vi "Main.vi"() -> ()   [LabVIEW 2020]
uses:
  <vilib>/Utility/miscctls.llb/LVBoundsTypeDef.ctl
  <vilib>/Utility/miscctls.llb/LVPointTypeDef.ctl
  <vilib>/Utility/miscctls.llb/LVRangeTypeDef.ctl
  <vilib>/DAQmx/read.llb/DAQmx Read (Analog 1D Wfm NChan NSamp).vi
  <vilib>/Waveform/WDTOps.llb/WDT Append Waveforms DBL.vi
  <vilib>/DAQmx/create/channels.llb/DAQmx Create Channel (AI-Voltage-Basic).vi
  <vilib>/DAQmx/configure/timing.llb/DAQmx Timing (Sample Clock).vi
  <vilib>/DAQmx/miscellaneous.llb/DAQmx Fill In Error Info.vi
  <vilib>/regexp/Match Regular Expression.xnode
  <resource>/objmgr/daqmx.rc
panel:
  out "Counter":dbl
  out "Continious Log Flag":bool
  in  "Continious Log":bool
  in  "Current Amplitude Range":dbl min=1.0 max=200.0 step=1.0
  in  "Voltage Amplitude Range":dbl min=1.0 max=1000.0 step=1.0
  in  "Experiment Name":string
  in  "Level Lower Limit, dB":dbl min=-200.0 max=-10.0 step=10.0
  in  "Freq Upper Limit, Hz":dbl min=0.0 step=1.0
  in  "Freq Lower Limit, Hz":dbl min=0.0 step=1.0
  out "Log flag":bool
  in  "Start Log":bool
  in  "Log length, sec":sgl min=0.2 max=600 step=0.1 format="%.1f"
  out "Current Spectrum":waveform(dbl)[](graph)
  out "Park Spectrum":waveform(dbl)[](graph)
  in  "Park Spectrum Button":bool
  in  "Current Spectrum Button":bool
  in  "Godograph Button":bool
  in  "Voltage Spectrum Button":bool
  in  "Current Button":bool
  in  "Voltage Button":bool
  in  "Plot length , sec":sgl min=0.2 max=60 step=0.1 format="%.1f"
  out "Voltage":waveform(dbl)[](graph)=[{"t0"=timestamp(3706707710.400176 s since 1904-01-01), "dt"=2.4999999999999957e-05, "Y"=array[8000 elements], "attributes"=variant("NI_ChannelName"=variant(string "Voltage A"), "NI_UnitDescription"=variant(string "Volts"))}, {"t0"=timestamp(3706707710.4001803 s since 1904-01-01), "dt"=2.4999999999999957e-05, "Y"=array[8000 elements], "attributes"=variant("NI_ChannelName"=variant(string "Voltage B"), "NI_UnitDescription"=variant(string "Volts"))}, {"t0"=timestamp(3706707710.4001846 s since 1904-01-01), "dt"=2.4999999999999957e-05, "Y"=array[8000 elements], "attributes"=variant("NI_ChannelName"=variant(string "Voltage C"), "NI_UnitDescription"=variant(string "Volts"))}]
  out "Current":waveform(dbl)[](graph)=[{"t0"=timestamp(3706707710.4001637 s since 1904-01-01), "dt"=2.4999999999999957e-05, "Y"=array[8000 elements], "attributes"=variant("NI_ChannelName"=variant(string "Current A"), "NI_UnitDescription"=variant(string "Volts"))}, {"t0"=timestamp(3706707710.400168 s since 1904-01-01), "dt"=2.4999999999999957e-05, "Y"=array[8000 elements], "attributes"=variant("NI_ChannelName"=variant(string "Current B"), "NI_UnitDescription"=variant(string "Volts"))}, {"t0"=timestamp(3706707710.4001718 s since 1904-01-01), "dt"=2.4999999999999957e-05, "Y"=array[8000 elements], "attributes"=variant("NI_ChannelName"=variant(string "Current C"), "NI_UnitDescription"=variant(string "Volts"))}]
  out "Voltage Spectrum":waveform(dbl)[](graph)
  out "Godograph":cluster{"Y":dbl[], "Y":dbl[]}[](graph)
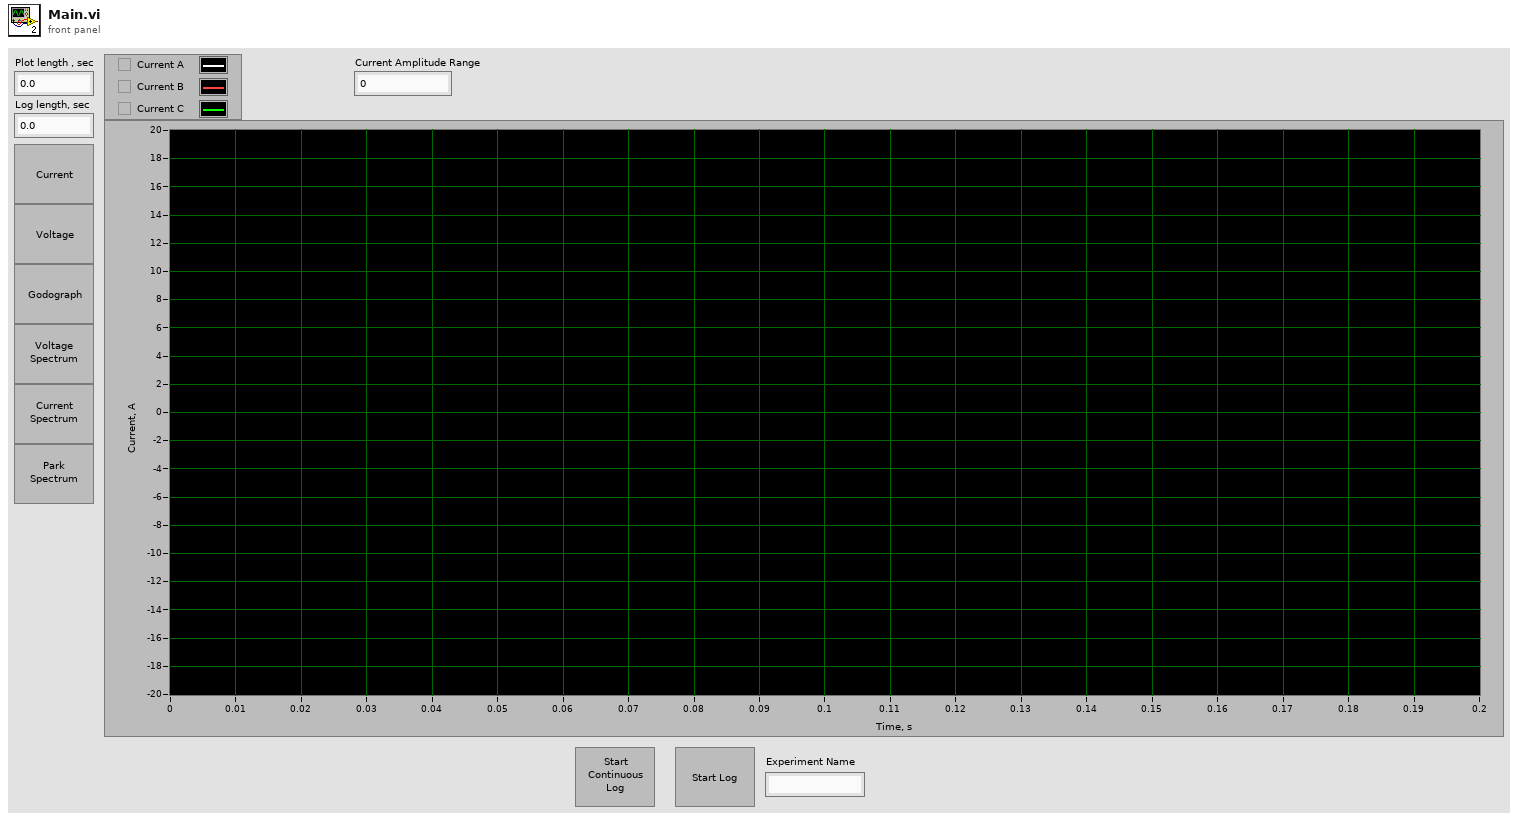
[diagram p1: front panel]
types:
  T1 = typedef "LVBoundsTypeDef.ctl" = cluster{"Width":u32, "Height":u32}
  T2 = typedef "LVPointTypeDef.ctl" = cluster{"Horizontal":i16, "Vertical":i16}
  T3 = enum16{"Always On", "Always Off", "Off While Running"}
  T4 = typedef "LVRangeTypeDef.ctl" = cluster{"Minimum":dbl, "Maximum":dbl, "Increment":dbl, "Minor Increment":dbl, "Start":dbl}
  T5 = enum8{"Enabled", "Disabled", "Disabled and Grayed Out"}
  T6 = enum16{"open", "open or create", "create or replace", "create", "open (read-only)"}
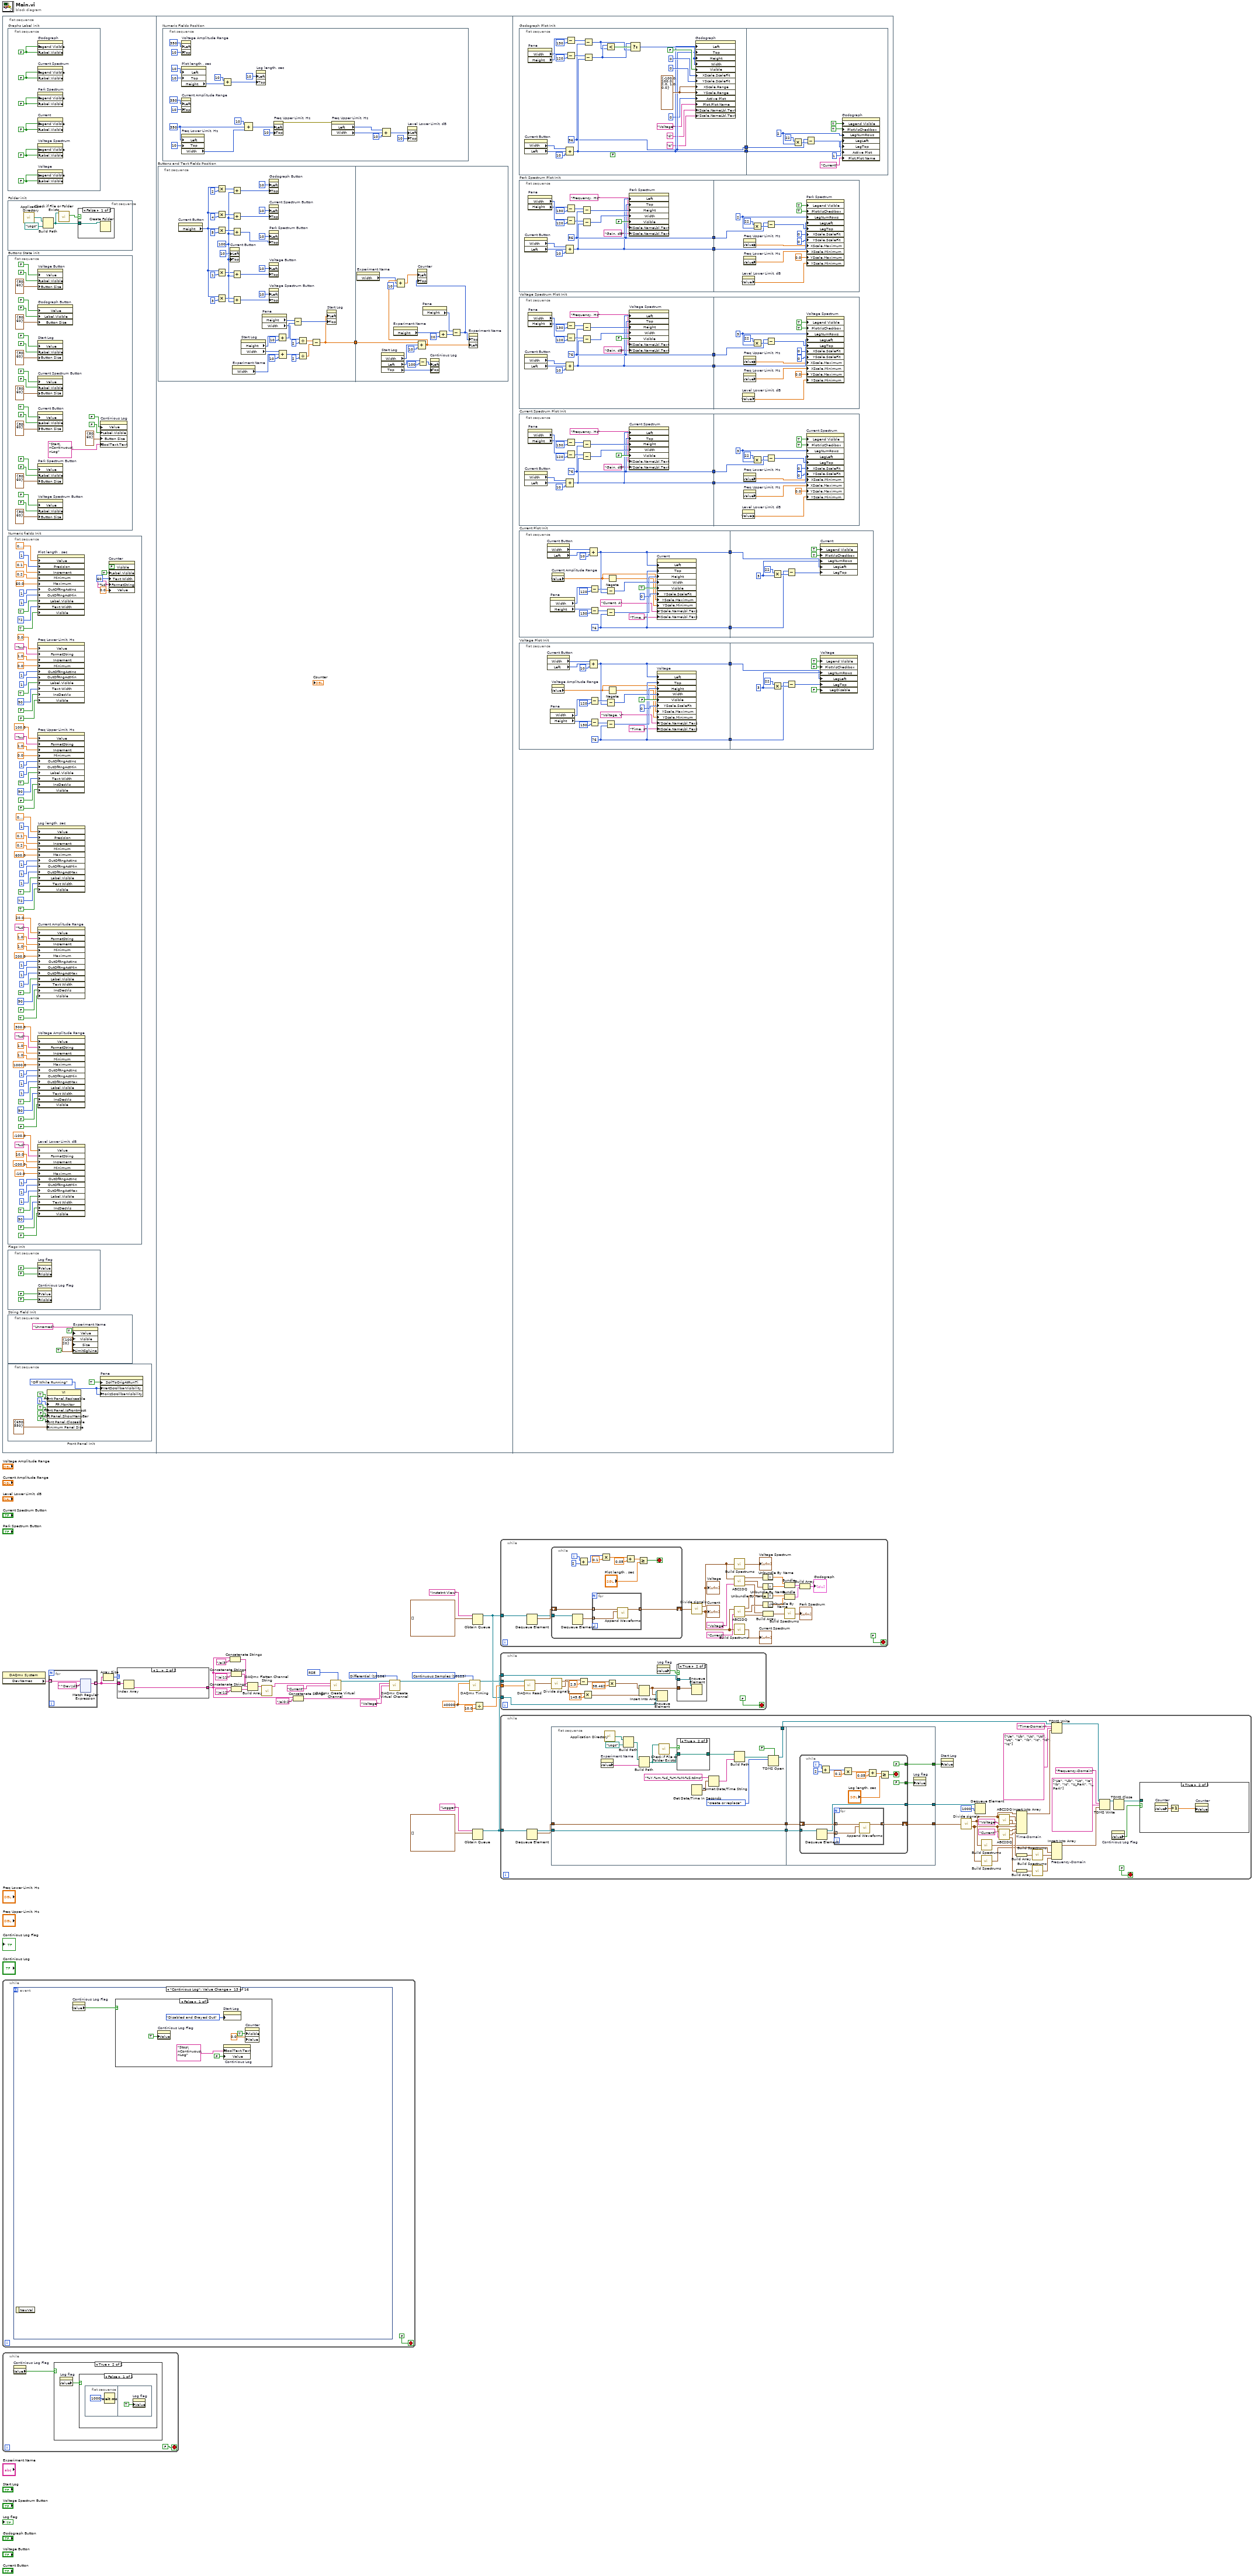
[diagram p0: block diagram]
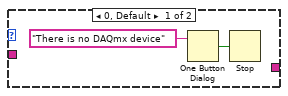
[diagram p2: hidden frame]
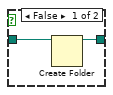
[diagram p6: hidden frame]
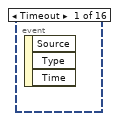
[diagram p8: hidden frame]
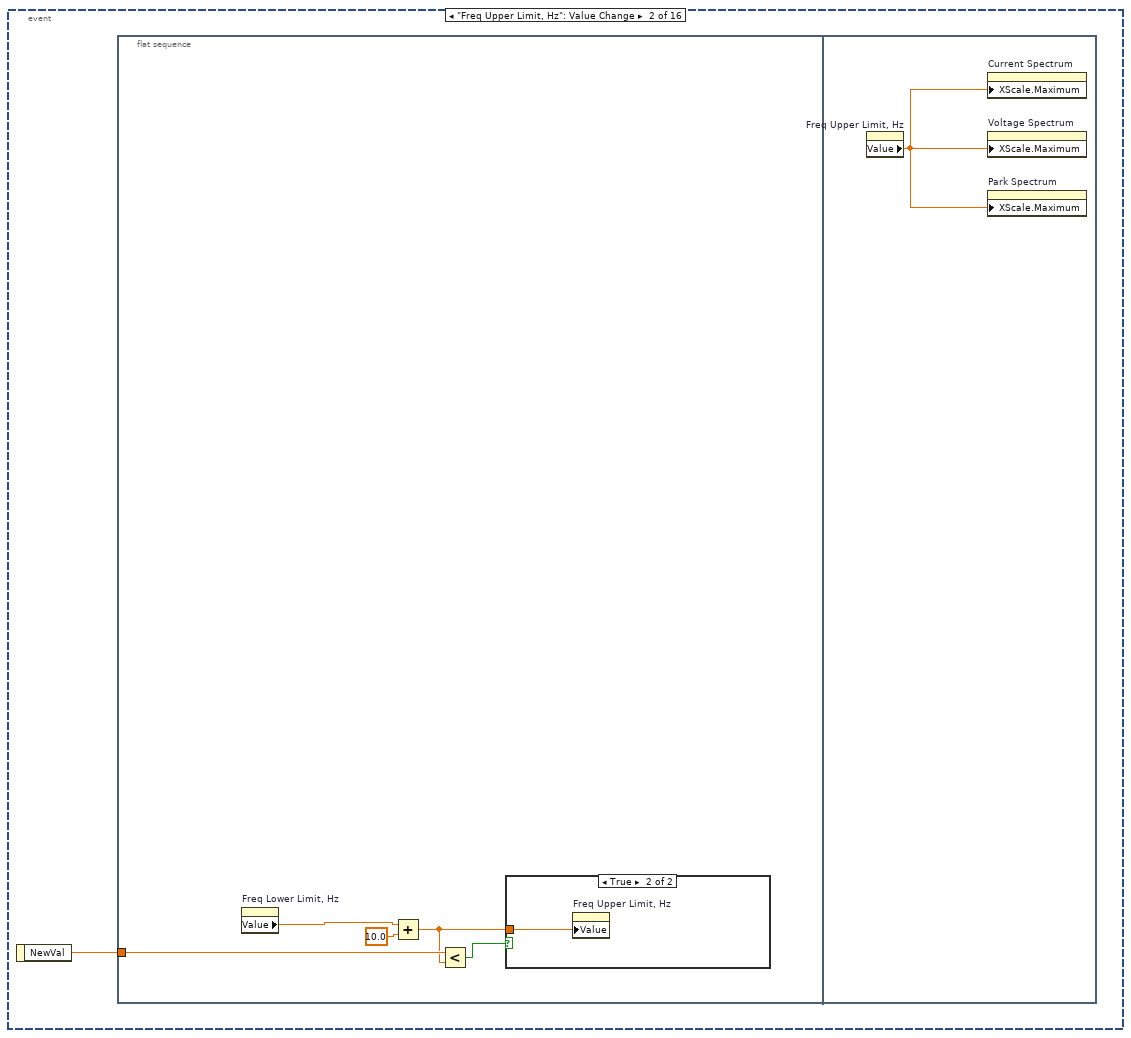
[diagram p9: hidden frame]
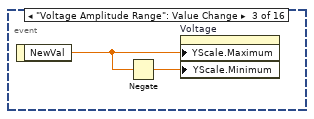
[diagram p11: hidden frame]
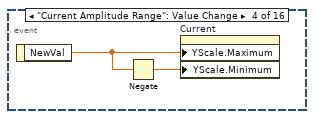
[diagram p12: hidden frame]
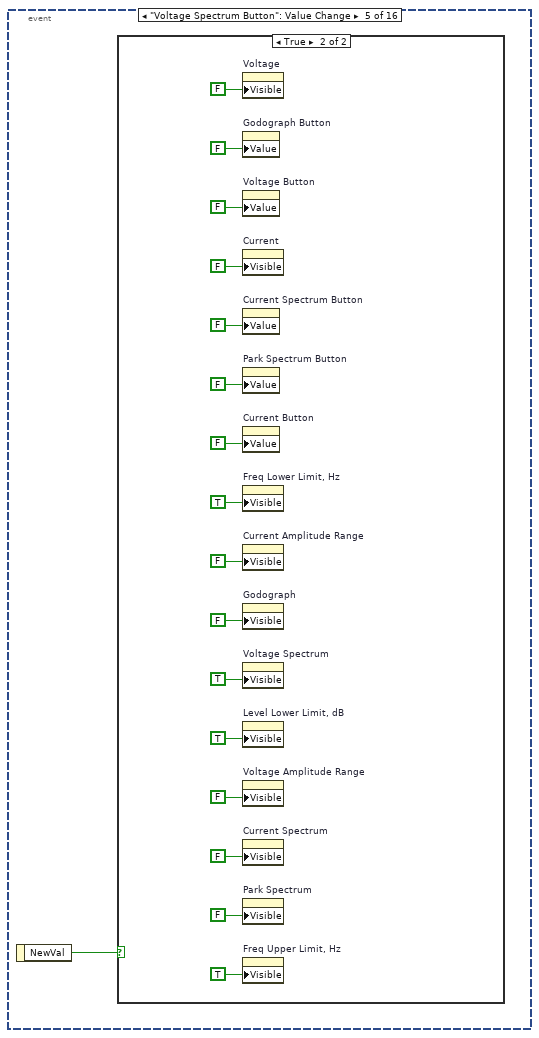
[diagram p13: hidden frame]
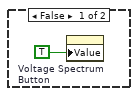
[diagram p14: hidden frame]
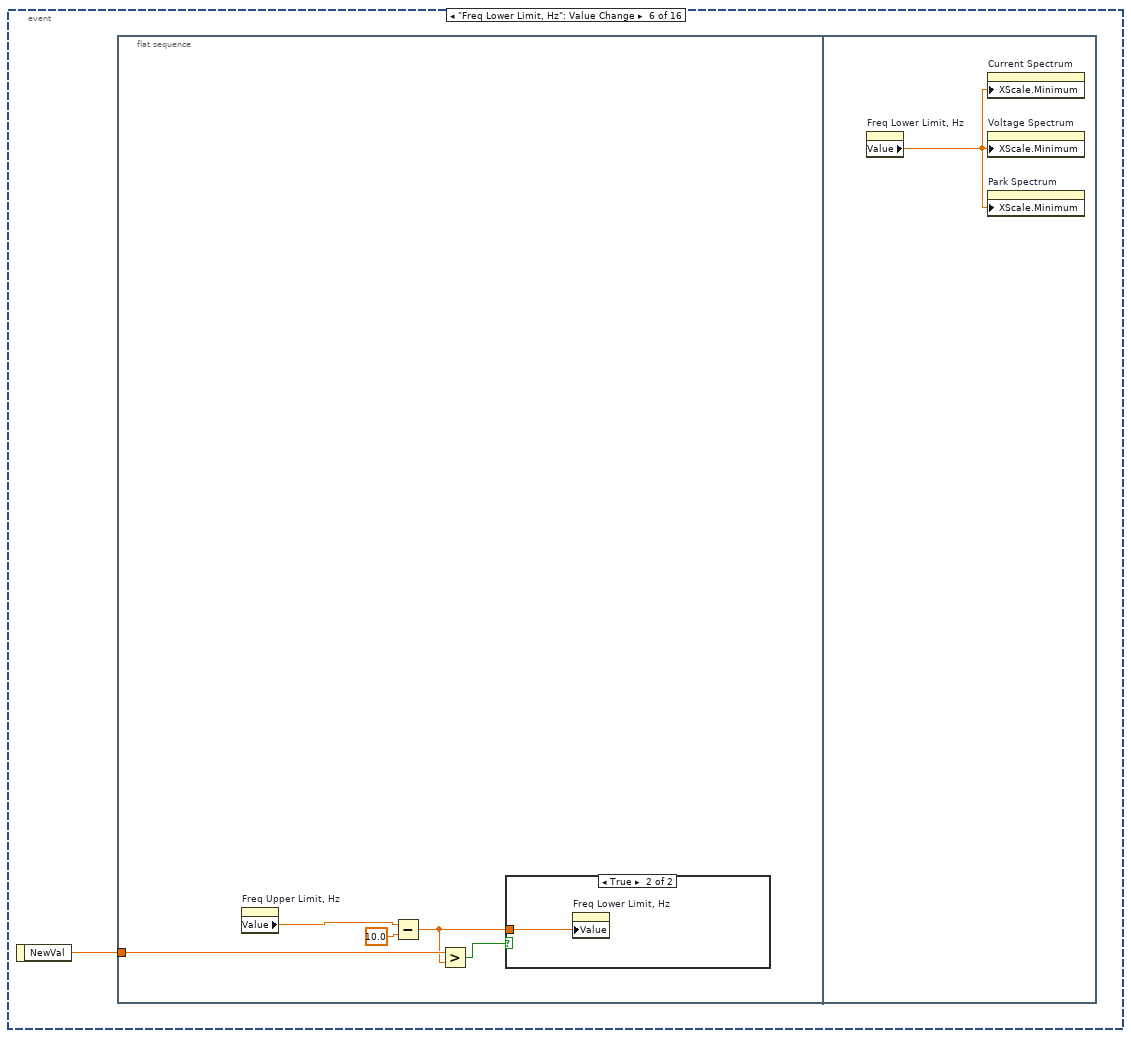
[diagram p15: hidden frame]
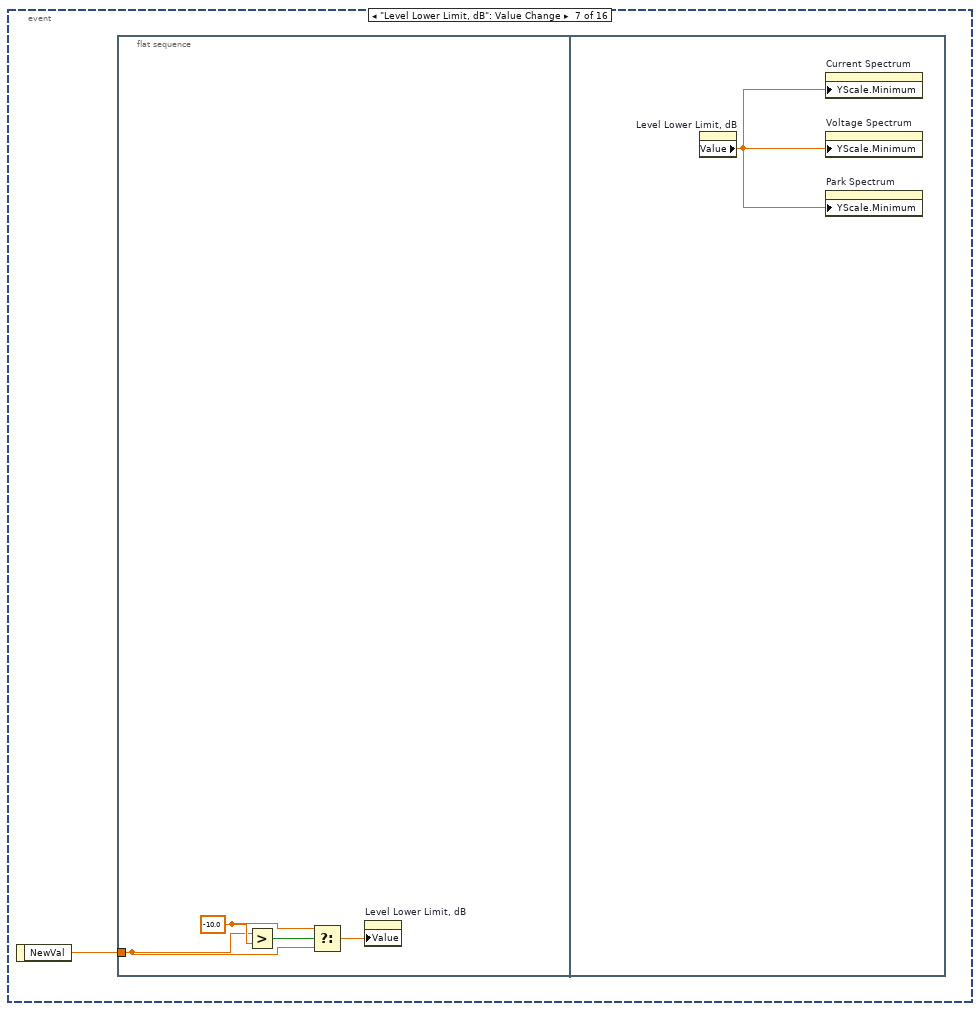
[diagram p17: hidden frame]
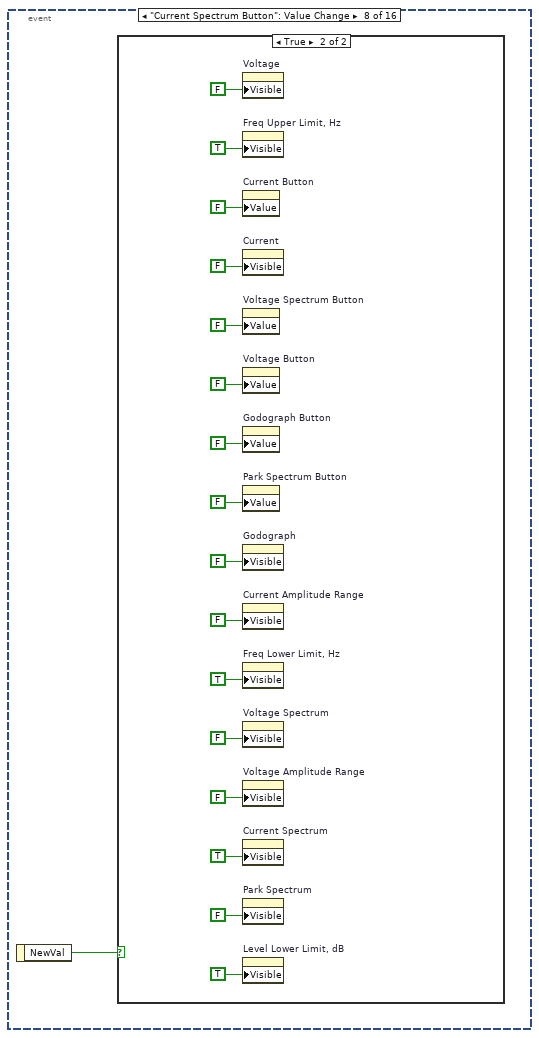
[diagram p18: hidden frame]
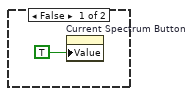
[diagram p19: hidden frame]
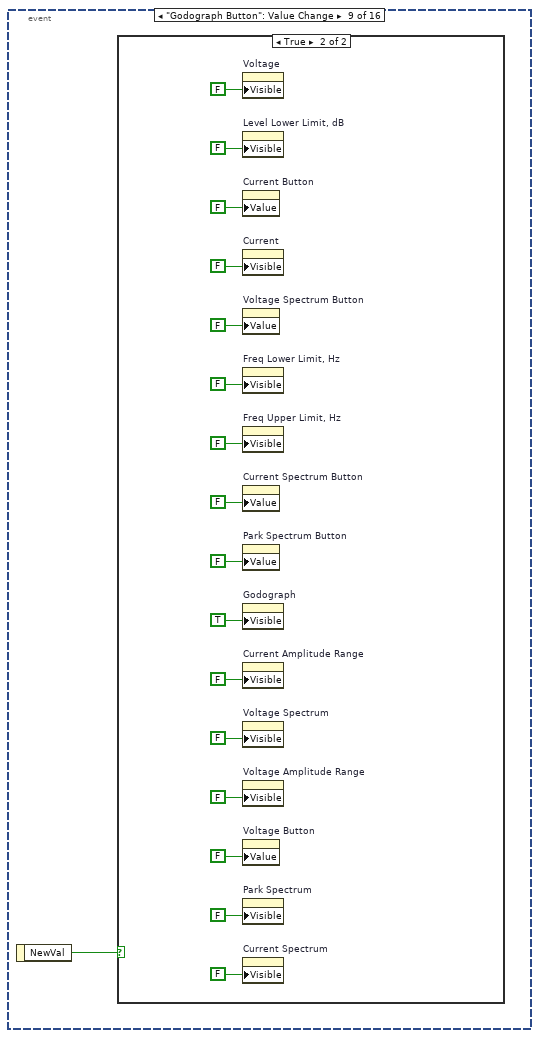
[diagram p20: hidden frame]
diagram:
  w16 = 40000.0 ("rate")
  w27 = 10123 items=["Finite Samples"=10178, "Continuous Samples"=10123, "Hardware Timed Single Point"=12522] ("sample mode")
  w30 = 10083 items=["Default"=-1, "RSE"=10083, "NRSE"=10078, "Differential"=10106, "Pseudodifferential"=12529] ("input terminal configuration")
  w31 = 10106 items=["Default"=-1, "RSE"=10083, "NRSE"=10078, "Differential"=10106, "Pseudodifferential"=12529] ("input terminal configuration")
  n1 = flat-sequence {
    frame #0 {
      n2 = flat-sequence "Graphs Label init" {
        frame #0 {
          w140 = FALSE ("Label.Visible")
          w139 = FALSE ("Label.Visible")
          w136 = FALSE ("Label.Visible")
          w137 = FALSE ("Legend:Visible")
          w138 = FALSE ("Legend:Visible")
          w135 = FALSE ("Legend:Visible")
          n3 = property on="Godograph" class="XYGraph (strict)"("Legend Visible"=w138, "Label.Visible"=w138) -> ()  [unwired: 2 in, 2 out]
          n4 = property on="Current Spectrum" class="WFGraph (strict)"("Legend Visible"=w139, "Label.Visible"=w139) -> ()  [unwired: 2 in, 2 out]
          n5 = property on="Park Spectrum" class="WFGraph (strict)"("Legend Visible"=w140, "Label.Visible"=w140) -> ()  [unwired: 2 in, 2 out]
          n6 = property on="Current" class="WFGraph (strict)"("Legend Visible"=w135, "Label.Visible"=w135) -> ()  [unwired: 2 in, 2 out]
          n7 = property on="Voltage Spectrum" class="WFGraph (strict)"("Legend Visible"=w136, "Label.Visible"=w136) -> ()  [unwired: 2 in, 2 out]
          n8 = property on="Voltage" class="WFGraph (strict)"("Legend Visible"=w137, "Label.Visible"=w137) -> ()  [unwired: 2 in, 2 out]
        }
      }
      n9 = flat-sequence "Folder init" {
        frame #0 {
          n10 = call <vilib>:"Application Directory.vi"() -> ("Application Directory"=w35:path)
          n11 = Build Path(base path=w35, name or relative path=path "Logs") -> (appended path=w32:path)
          n12 = call <vilib>:"Check if File or Folder Exists.vi"("path"=w32) -> ("file or folder exists?"=w33:bool)  [unwired: 8 in, 2 out]
          n13 = case shown="False" w33 {
            tunnel: w32 -> [w36 _]
            frame False {
              n14 = Create Folder(path (use dialog)=w36) -> ()  [unwired: 2 in, 3 out]
            }
            frame True {
            }
          }
        }
      }
      n15 = flat-sequence "Buttons State init" {
        frame #0 {
          n16 = property on="Voltage Button" class="Bool (strict)"("Value"=FALSE ("Current Button"), "Label.Visible"=FALSE, "Button Size"=T1 {"Width"=80, "Height"=60}) -> ()  [unwired: 2 in, 2 out]
          n17 = property on="Godograph Button" class="Bool (strict)"("Value"=FALSE ("Current Button"), "Label.Visible"=FALSE, "Button Size"=T1 {"Width"=80, "Height"=60} ("XControl:Container Bounds")) -> ()  [unwired: 2 in, 2 out]
          n18 = property on="Start Log" class="Bool (strict)"("Value"=FALSE ("Start Log"), "Label.Visible"=FALSE, "Button Size"=T1 {"Width"=80, "Height"=60}) -> ()  [unwired: 2 in, 2 out]
          n19 = property on="Current Spectrum Button" class="Bool (strict)"("Value"=FALSE ("Current Button"), "Label.Visible"=FALSE, "Button Size"=T1 {"Width"=80, "Height"=60}) -> ()  [unwired: 2 in, 2 out]
          n20 = property on="Current Button" class="Bool (strict)"("Value"=TRUE ("Current Button"), "Label.Visible"=FALSE, "Button Size"=T1 {"Width"=80, "Height"=60}) -> ()  [unwired: 2 in, 2 out]
          n21 = property on="Park Spectrum Button" class="Bool (strict)"("Value"=FALSE ("Current Button"), "Label.Visible"=FALSE, "Button Size"=T1 {"Width"=80, "Height"=60}) -> ()  [unwired: 2 in, 2 out]
          n22 = property on="Voltage Spectrum Button" class="Bool (strict)"("Value"=FALSE ("Current Button"), "Label.Visible"=FALSE ("Value (Signaling)"), "Button Size"=T1 {"Width"=80, "Height"=60}) -> ()  [unwired: 2 in, 2 out]
          n23 = property on="Continious Log" class="Bool (strict)"("Value"=FALSE ("Start Log"), "Label.Visible"=FALSE, "Button Size"=T1 {"Width"=80, "Height"=60}, "BoolText.Text"="Start\nContinuous\nLog" ("Boolean Text.Text")) -> ()  [unwired: 2 in, 2 out]
        }
      }
      n24 = flat-sequence "Numeric fields Init" {
        frame #0 {
          n25 = property on="Plot length , sec" class="DigNum (strict)"("Value"=sgl 0.2 ("Plot length , sec"), "Precision"=u8 1 ("Display Format:Precision"), "Increment"=0.1 ("Data Entry Limits:Increment"), "Minimum"=0.2 ("Data Entry Limits:Minimum"), "Maximum"=60.0 ("Data Entry Limits:Maximum"), "OutOfRngActInc"=u8 1 ("Response to Value Outside Limits:Increment"), "OutOfRngActMin"=u8 1 ("Response to Value Outside Limits:Minimum"), "Label.Visible"=TRUE, "Text Width"=u32 72, "Visible"=TRUE) -> ()  [unwired: 2 in, 2 out]
          n26 = property on="Freq Lower Limit, Hz" class="DigNum (strict)"("Value"=0.0 ("Lower Limit"), "FormatString"="%u" ("Format String"), "Increment"=1.0 ("Data Entry Limits:Increment"), "Minimum"=0.0 ("Data Entry Limits:Minimum"), "OutOfRngActInc"=u8 1 ("Response to Value Outside Limits:Increment"), "OutOfRngActMin"=u8 1 ("Response to Value Outside Limits:Minimum"), "Label.Visible"=TRUE, "Text Width"=u32 90, "IncDecVis"=FALSE ("Increment/Decrement Visible?"), "Visible"=FALSE) -> ()  [unwired: 2 in, 2 out]
          n27 = property on="Freq Upper Limit, Hz" class="DigNum (strict)"("Value"=100.0 ("Lower Limit"), "FormatString"="%u" ("Format String"), "Increment"=1.0 ("Data Entry Limits:Increment"), "Minimum"=0.0 ("Data Entry Limits:Minimum"), "OutOfRngActInc"=u8 1 ("Response to Value Outside Limits:Increment"), "OutOfRngActMin"=u8 1 ("Response to Value Outside Limits:Minimum"), "Label.Visible"=TRUE, "Text Width"=u32 90, "IncDecVis"=FALSE ("Increment/Decrement Visible?"), "Visible"=FALSE) -> ()  [unwired: 2 in, 2 out]
          n28 = property on="Log length, sec" class="DigNum (strict)"("Value"=sgl 0.2 ("Plot length , sec"), "Precision"=u8 1 ("Display Format:Precision"), "Increment"=0.1 ("Data Entry Limits:Increment"), "Minimum"=0.2 ("Data Entry Limits:Minimum"), "Maximum"=600.0 ("Data Entry Limits:Minimum"), "OutOfRngActInc"=u8 1 ("Response to Value Outside Limits:Increment"), "OutOfRngActMin"=u8 1 ("Response to Value Outside Limits:Minimum"), "OutOfRngActMax"=u8 1 ("Response to Value Outside Limits:Maximum"), "Label.Visible"=TRUE, "Text Width"=u32 72, "Visible"=TRUE) -> ()  [unwired: 2 in, 2 out]
          n29 = property on="Current Amplitude Range" class="DigNum (strict)"("Value"=20.0 ("Lower Limit"), "FormatString"="%d" ("Format String"), "Increment"=1.0 ("Data Entry Limits:Increment"), "Minimum"=1.0 ("Data Entry Limits:Minimum"), "Maximum"=200.0 ("Data Entry Limits:Maximum"), "OutOfRngActInc"=u8 1 ("Response to Value Outside Limits:Increment"), "OutOfRngActMin"=u8 1 ("Response to Value Outside Limits:Minimum"), "OutOfRngActMax"=u8 1 ("Response to Value Outside Limits:Maximum"), "Label.Visible"=TRUE, "Text Width"=u32 90, "IncDecVis"=FALSE ("Increment/Decrement Visible?"), "Visible"=TRUE) -> ()  [unwired: 2 in, 2 out]
          n30 = property on="Voltage Amplitude Range" class="DigNum (strict)"("Value"=300.0 ("Lower Limit"), "FormatString"="%d" ("Format String"), "Increment"=1.0 ("Data Entry Limits:Increment"), "Minimum"=1.0 ("Data Entry Limits:Minimum"), "Maximum"=1000.0 ("Data Entry Limits:Maximum"), "OutOfRngActInc"=u8 1 ("Response to Value Outside Limits:Increment"), "OutOfRngActMin"=u8 1 ("Response to Value Outside Limits:Minimum"), "OutOfRngActMax"=u8 1 ("Response to Value Outside Limits:Maximum"), "Label.Visible"=TRUE, "Text Width"=u32 90, "IncDecVis"=FALSE ("Increment/Decrement Visible?"), "Visible"=FALSE) -> ()  [unwired: 2 in, 2 out]
          n31 = property on="Level Lower Limit, dB" class="DigNum (strict)"("Value"=-100.0 ("Lower Limit"), "FormatString"="%d" ("Format String"), "Increment"=10.0 ("Data Entry Limits:Increment"), "Minimum"=-200.0 ("Data Entry Limits:Minimum"), "Maximum"=-10.0 ("Data Entry Limits:Maximum"), "OutOfRngActInc"=u8 1 ("Response to Value Outside Limits:Increment"), "OutOfRngActMin"=u8 1 ("Response to Value Outside Limits:Minimum"), "OutOfRngActMax"=u8 1 ("Response to Value Outside Limits:Maximum"), "Label.Visible"=TRUE, "Text Width"=u32 90, "IncDecVis"=FALSE ("Increment/Decrement Visible?"), "Visible"=FALSE) -> ()  [unwired: 2 in, 2 out]
          n32 = property on="Counter" class="DigNum (strict)"("Visible"=FALSE, "Label.Visible"=TRUE, "Text Width"=u32 60 ("Numeric Text.Size:Height"), "FormatString"="%d" ("Format String"), "Value"=0.0 ("Counter")) -> ()  [unwired: 2 in, 2 out]
        }
      }
      n33 = flat-sequence "Flags Init" {
        frame #0 {
          n34 = property on="Log flag" class="Bool (strict)"("Value"=FALSE ("Log flag"), "Visible"=FALSE) -> ()  [unwired: 2 in, 2 out]
          n35 = property on="Continious Log Flag" class="Bool (strict)"("Value"=FALSE ("Log flag"), "Visible"=FALSE) -> ()  [unwired: 2 in, 2 out]
        }
      }
      n36 = flat-sequence "String Field Init" {
        frame #0 {
          n37 = property on="Experiment Name" class="Str"("Value"="Unnamed" ("Experiment Name"), "Visible"=TRUE, "Size"=T1 {"Width"=100, "Height"=20}, "LimitSglLine"=TRUE ("Limit To Single Line?")) -> ()  [unwired: 2 in, 2 out]
        }
      }
      n38 = flat-sequence "Front Panel Init" {
        frame #0 {
          w133 = T3."Off While Running" ("Vertical Scrollbar Visibility")
          n39 = property class="VI"("Front Panel.Resizeable"=TRUE ("Front Panel Window:Resizable"), "FP.Monitor"=u16 1 ("Front Panel Window:Monitor"), "Front Panel.IsFrontmost"=TRUE ("Front Panel Window:Is Frontmost"), "Front Panel.ShowMenuBar"=FALSE ("Front Panel Window:Show Menu Bar"), "Front Panel.Closeable"=FALSE ("Front Panel Window:Closeable"), "Minimum Panel Size"=T2 {"Horizontal"=650, "Vertical"=550} ("Front Panel Window:Minimum Size")) -> ()  [unwired: 2 in, 2 out]
          n40 = property on="Pane" class="Pane"("ScrlToOrigAtRunTi"=TRUE ("Scroll To Origin At Run Time"), "VertScrollbarVisibility"=w133, "HorizScrollbarVisibility"=w133) -> ()  [unwired: 2 in, 2 out]
        }
      }
    }
    frame #1 {
      n41 = flat-sequence "Buttons and Text Fields Position" {
        tunnel: [w189] -> w166
        tunnel: w166 -> [w238]
        frame #0 {
          w207 = 100 ("Position:Top")
          n42 = property on="Current Button" class="Bool (strict)"() -> ("Height"=w205:u32)  [unwired: 2 in, 2 out]
          n43 = Multiply(x=w205, y=u32 2) -> (x*y=w221:u32)
          n44 = Multiply(x=w205, y=u32 4) -> (x*y=w213:u32)
          n45 = Multiply(x=w205, y=u32 5) -> (x*y=w210:u32)
          n46 = Multiply(x=w205, y=u32 1) -> (x*y=w204:u32)
          n47 = Multiply(x=w205, y=u32 3) -> (x*y=w218:u32)
          n48 = property on="Current Button" class="Bool (strict)"("Left"=10 ("Position:Left"), "Top"=w207) -> ()  [unwired: 2 in, 2 out]
          n49 = Add(x=w221, y=w207) -> (x+y=w223:u32)
          n50 = Add(x=w213, y=w207) -> (x+y=w215:u32)
          n51 = Add(x=w210, y=w207) -> (x+y=w208:u32)
          n52 = Add(x=w204, y=w207) -> (x+y=w224:u32)
          n53 = Add(x=w218, y=w207) -> (x+y=w216:u32)
          n54 = property on="Experiment Name" class="Str"() -> ("Width"=w192:u32)  [unwired: 2 in, 2 out]
          n55 = property on="Start Log" class="Bool (strict)"() -> ("Height"=w203:u32, "Width"=w193:u32)  [unwired: 2 in, 2 out]
          n56 = property on="Pane" class="Pane"() -> ("Height"=w201:u32, "Width"=w196:u32)  [unwired: 2 in, 2 out]
          n57 = property on="Godograph Button" class="Bool (strict)"("Left"=10 ("Position:Left"), "Top"=w223) -> ()  [unwired: 2 in, 2 out]
          n58 = property on="Current Spectrum Button" class="Bool (strict)"("Left"=10 ("Position:Left"), "Top"=w215) -> ()  [unwired: 2 in, 2 out]
          n59 = property on="Park Spectrum Button" class="Bool (strict)"("Left"=10 ("Position:Left"), "Top"=w208) -> ()  [unwired: 2 in, 2 out]
          n60 = property on="Voltage Button" class="Bool (strict)"("Left"=10 ("Position:Left"), "Top"=w224) -> ()  [unwired: 2 in, 2 out]
          n61 = property on="Voltage Spectrum Button" class="Bool (strict)"("Left"=10 ("Position:Left"), "Top"=w216) -> ()  [unwired: 2 in, 2 out]
          n62 = Add(x=w203, y=u32 10) -> (x+y=w200:u32)
          n63 = Compound Arithmetic op=ADD(w193, w192, u32 10 ("value")) -> (w190:u32)
          n64 = Subtract(x=w201, y=w200) -> (x-y=w199:u32)
          n65 = Divide(x=w196, y=u32 2) -> (x/y=w195:dbl)
          n66 = Divide(x=w190, y=u32 2) -> (x/y=w194:dbl)
          n67 = Subtract(x=w195, y=w194) -> (x-y=w189:dbl)
          n68 = property on="Start Log" class="Bool (strict)"("Left"=w189, "Top"=w199) -> ()  [unwired: 2 in, 2 out]
        }
        frame #1 {
          n69 = property on="Experiment Name" class="Str"() -> ("Width"=w229:u32)  [unwired: 2 in, 2 out]
          n70 = property on="Start Log" class="Bool (strict)"() -> ("Width"=w237:u32, "Left"=w234:i32, "Top"=w235:i32)  [unwired: 2 in, 2 out]
          n71 = property on="Experiment Name" class="Str"() -> ("Height"=w240:u32)  [unwired: 2 in, 2 out]
          n72 = Subtract(x=w234, y=100) -> (x-y=w232:i32)
          n73 = Compound Arithmetic op=ADD(w238, w237, u32 10 ("value")) -> (w230:dbl)
          n74 = Compound Arithmetic op=ADD(w230, w229, u32 10 ("value")) -> (w227:dbl)
          n75 = property on="Pane" class="Pane"() -> ("Height"=w241:u32)  [unwired: 2 in, 2 out]
          n76 = property on="Continious Log" class="Bool (strict)"("Left"=w232, "Top"=w235) -> ()  [unwired: 2 in, 2 out]
          n77 = Add(x=w240, y=u32 20) -> (x+y=w242:u32)
          n78 = Subtract(x=w241, y=w242) -> (x-y=w231:u32)
          n79 = property on="Counter" class="DigNum (strict)"("Left"=w227, "Top"=w231) -> ()  [unwired: 2 in, 2 out]
          n80 = property on="Experiment Name" class="Str"("Top"=w231, "Left"=w230) -> ()  [unwired: 2 in, 2 out]
        }
      }
      n81 = flat-sequence "Numeric Fields Position" {
        frame #0 {
          w178 = 350 ("Position:Left")
          n82 = property on="Voltage Amplitude Range" class="DigNum (strict)"("Left"=350 ("Position:Left"), "Top"=10 ("Position:Top")) -> ()  [unwired: 2 in, 2 out]
          n83 = property on="Plot length , sec" class="DigNum (strict)"("Left"=10 ("Position:Left"), "Top"=10 ("Position:Top")) -> ("Height"=w184:u32)  [unwired: 2 in, 2 out]
          n84 = property on="Current Amplitude Range" class="DigNum (strict)"("Left"=350 ("Position:Left"), "Top"=10 ("Position:Top")) -> ()  [unwired: 2 in, 2 out]
          n85 = property on="Freq Lower Limit, Hz" class="DigNum (strict)"("Left"=w178, "Top"=10 ("Position:Top")) -> ("Width"=w179:u32)  [unwired: 2 in, 2 out]
          n86 = Add(x=10 ("Position:Top"), y=w184) -> (x+y=w183:u32)
          n87 = Compound Arithmetic op=ADD(10 ("value"), w178, w179) -> (w180:u32)
          n88 = property on="Log length, sec" class="DigNum (strict)"("Left"=10 ("Position:Left"), "Top"=w183) -> ()  [unwired: 2 in, 2 out]
          n89 = property on="Freq Upper Limit, Hz" class="DigNum (strict)"("Left"=w180, "Top"=10 ("Position:Left")) -> (error out=w171:errorcluster)  [unwired: 2 in, 1 out]
          n90 = property on="Freq Upper Limit, Hz" class="DigNum (strict)"(error in=w171) -> ("Left"=w176:i32, "Width"=w175:u32)  [unwired: 1 in, 2 out]
          n91 = Compound Arithmetic op=ADD(w176, w175, u32 10 ("value")) -> (w172:u32)
          n92 = property on="Level Lower Limit, dB" class="DigNum (strict)"("Left"=w172, "Top"=10 ("Position:Top")) -> ()  [unwired: 2 in, 2 out]
        }
      }
    }
    frame #2 {
      n93 = flat-sequence "Godograph Plot Init" {
        tunnel: [w290] -> w254
        tunnel: [w289] -> w253
        tunnel: w254 -> [w315]
        tunnel: w253 -> [w311]
        frame #0 {
          w291 = T4 {"Minimum"=-100.0, "Maximum"=100.0, "Increment"=2.0, "Minor Increment"=1.0, "Start"=0.0} ("Y Scale.Range")
          (unwired) FALSE ("Visible")
          w289 = 56 ("Position:Top")
          n94 = property on="Current Button" class="Bool (strict)"() -> ("Width"=w307:u32, "Left"=w306:i32)  [unwired: 2 in, 2 out]
          n95 = property on="Pane" class="Pane"() -> ("Width"=w299:u32, "Height"=w296:u32)  [unwired: 2 in, 2 out]
          n96 = Subtract(x=w296, y=u32 130) -> (x-y=w302:u32)
          n97 = Subtract(x=w299, y=u32 120) -> (x-y=w303:u32)
          n98 = Compound Arithmetic op=ADD(w307, w306, 10 ("value")) -> (w290:u32)
          n99 = Subtract(x=w302, y=w289) -> (x-y=w295:u32)
          n100 = Subtract(x=w303, y=w290) -> (x-y=w297:u32)
          n101 = Less?(x=w297, y=w295) -> (x < y?=w300:bool)
          n102 = Select(t=w297, s=w300, f=w295) -> (s? t:f=w298:u32)
          n103 = property on="Godograph" class="XYGraph (strict)"("Left"=w290, "Top"=w289, "Height"=w298, "Width"=w298, "Visible"=FALSE, "XScale.ScaleFit"=u8 0 ("X Scale.Scale Fit"), "YScale.ScaleFit"=u8 0 ("Y Scale.Scale Fit"), "XScale.Range"=w291, "YScale.Range"=w291, "Active Plot"=u32 0, "Plot.Plot Name"="Voltage", "XScale.NameLbl.Text"="d" ("X Scale.Name Label.Text"), "YScale.NameLbl.Text"="q" ("Y Scale.Name Label.Text")) -> ()  [unwired: 2 in, 2 out]
        }
        frame #1 {
          w313 = u32 2 ("Legend:Number of Rows")
          n104 = Multiply(x=i8 22, y=w313) -> (x*y=w312:u32)
          n105 = Subtract(x=w311, y=w312) -> (x-y=w310:u32)
          n106 = property on="Godograph" class="XYGraph (strict)"("Legend Visible"=TRUE ("Legend:Visible"), "PlotVisCheckbox"=TRUE ("Legend:Plot Visibility Checkbox Visible"), "LegNumRows"=w313, "LegLeft"=w315, "LegTop"=w310, "Active Plot"=u32 1, "Plot.Plot Name"="Current") -> ()  [unwired: 2 in, 2 out]
        }
      }
      n107 = flat-sequence "Park Spectrum Plot Init" {
        tunnel: [w258] -> w252
        tunnel: [w257] -> w251
        tunnel: w252 -> [w278]
        tunnel: w251 -> [w277]
        frame #0 {
          w258 = 56 ("Position:Top")
          n108 = property on="Current Button" class="Bool (strict)"() -> ("Width"=w270:u32, "Left"=w269:i32)  [unwired: 2 in, 2 out]
          n109 = property on="Pane" class="Pane"() -> ("Width"=w267:u32, "Height"=w259:u32)  [unwired: 2 in, 2 out]
          n110 = Subtract(x=w259, y=u32 130) -> (x-y=w264:u32)
          n111 = Subtract(x=w267, y=u32 120) -> (x-y=w265:u32)
          n112 = Compound Arithmetic op=ADD(w270, w269, 10 ("value")) -> (w257:u32)
          n113 = Subtract(x=w264, y=w258) -> (x-y=w262:u32)
          n114 = Subtract(x=w265, y=w257) -> (x-y=w261:u32)
          n115 = property on="Park Spectrum" class="WFGraph (strict)"("Left"=w257, "Top"=w258, "Height"=w262, "Width"=w261, "Visible"=FALSE, "XScale.NameLbl.Text"="Frequency, Hz" ("X Scale.Name Label.Text"), "YScale.NameLbl.Text"="Gain, dB" ("Y Scale.Name Label.Text")) -> ()  [unwired: 2 in, 2 out]
        }
        frame #1 {
          w281 = u32 2 ("Legend:Number of Rows")
          n116 = property on="Level Lower Limit, dB" class="DigNum (strict)"() -> ("Value"=w271:dbl)  [unwired: 2 in, 2 out]
          n117 = property on="Freq Upper Limit, Hz" class="DigNum (strict)"() -> ("Value"=w274:dbl)  [unwired: 2 in, 2 out]
          n118 = property on="Freq Lower Limit, Hz" class="DigNum (strict)"() -> ("Value"=w275:dbl)  [unwired: 2 in, 2 out]
          n119 = Multiply(x=i8 22, y=w281) -> (x*y=w280:u32)
          n120 = Subtract(x=w278, y=w280) -> (x-y=w279:u32)
          n121 = property on="Park Spectrum" class="WFGraph (strict)"("Legend Visible"=TRUE ("Legend:Visible"), "PlotVisCheckbox"=TRUE ("Legend:Plot Visibility Checkbox Visible"), "LegNumRows"=w281, "LegLeft"=w277, "LegTop"=w279, "XScale.ScaleFit"=u8 0 ("X Scale.Scale Fit"), "YScale.ScaleFit"=u8 0 ("Y Scale.Scale Fit"), "XScale.Maximum"=w274, "XScale.Minimum"=w275, "YScale.Maximum"=0.0 ("Y Scale.Range:Maximum"), "YScale.Minimum"=w271) -> ()  [unwired: 2 in, 2 out]
        }
      }
      n122 = flat-sequence "Voltage Spectrum Plot Init" {
        tunnel: [w351] -> w250
        tunnel: [w350] -> w249
        tunnel: w250 -> [w371]
        tunnel: w249 -> [w370]
        frame #0 {
          w351 = 76 ("Position:Top")
          n123 = property on="Current Button" class="Bool (strict)"() -> ("Width"=w363:u32, "Left"=w362:i32)  [unwired: 2 in, 2 out]
          n124 = property on="Pane" class="Pane"() -> ("Width"=w360:u32, "Height"=w352:u32)  [unwired: 2 in, 2 out]
          n125 = Subtract(x=w352, y=u32 130) -> (x-y=w357:u32)
          n126 = Subtract(x=w360, y=u32 120) -> (x-y=w358:u32)
          n127 = Compound Arithmetic op=ADD(w363, w362, 10 ("value")) -> (w350:u32)
          n128 = Subtract(x=w357, y=w351) -> (x-y=w355:u32)
          n129 = Subtract(x=w358, y=w350) -> (x-y=w354:u32)
          n130 = property on="Voltage Spectrum" class="WFGraph (strict)"("Left"=w350, "Top"=w351, "Height"=w355, "Width"=w354, "Visible"=FALSE, "XScale.NameLbl.Text"="Frequency, Hz" ("X Scale.Name Label.Text"), "YScale.NameLbl.Text"="Gain, dB" ("Y Scale.Name Label.Text")) -> ()  [unwired: 2 in, 2 out]
        }
        frame #1 {
          w374 = u32 3 ("Legend:Number of Rows")
          n131 = property on="Level Lower Limit, dB" class="DigNum (strict)"() -> ("Value"=w365:dbl)  [unwired: 2 in, 2 out]
          n132 = property on="Freq Upper Limit, Hz" class="DigNum (strict)"() -> ("Value"=w367:dbl)  [unwired: 2 in, 2 out]
          n133 = property on="Freq Lower Limit, Hz" class="DigNum (strict)"() -> ("Value"=w368:dbl)  [unwired: 2 in, 2 out]
          n134 = Multiply(x=i8 22, y=w374) -> (x*y=w373:u32)
          n135 = Subtract(x=w371, y=w373) -> (x-y=w372:u32)
          n136 = property on="Voltage Spectrum" class="WFGraph (strict)"("Legend Visible"=TRUE ("Legend:Visible"), "PlotVisCheckbox"=TRUE ("Legend:Plot Visibility Checkbox Visible"), "LegNumRows"=w374, "LegLeft"=w370, "LegTop"=w372, "XScale.ScaleFit"=u8 0 ("X Scale.Scale Fit"), "YScale.ScaleFit"=u8 0 ("Y Scale.Scale Fit"), "XScale.Maximum"=w367, "XScale.Minimum"=w368, "YScale.Maximum"=0.0 ("Y Scale.Range:Maximum"), "YScale.Minimum"=w365) -> ()  [unwired: 2 in, 2 out]
        }
      }
      n137 = flat-sequence "Current Spectrum Plot Init" {
        tunnel: [w321] -> w248
        tunnel: [w320] -> w247
        tunnel: w248 -> [w341]
        tunnel: w247 -> [w340]
        frame #0 {
          w320 = 76 ("Position:Top")
          n138 = property on="Current Button" class="Bool (strict)"() -> ("Width"=w333:u32, "Left"=w332:i32)  [unwired: 2 in, 2 out]
          n139 = property on="Pane" class="Pane"() -> ("Width"=w330:u32, "Height"=w322:u32)  [unwired: 2 in, 2 out]
          n140 = Subtract(x=w322, y=u32 130) -> (x-y=w327:u32)
          n141 = Subtract(x=w330, y=u32 120) -> (x-y=w328:u32)
          n142 = Compound Arithmetic op=ADD(w333, w332, 10 ("value")) -> (w321:u32)
          n143 = Subtract(x=w327, y=w320) -> (x-y=w325:u32)
          n144 = Subtract(x=w328, y=w321) -> (x-y=w324:u32)
          n145 = property on="Current Spectrum" class="WFGraph (strict)"("Left"=w321, "Top"=w320, "Height"=w325, "Width"=w324, "Visible"=FALSE, "XScale.NameLbl.Text"="Frequency, Hz" ("X Scale.Name Label.Text"), "YScale.NameLbl.Text"="Gain, dB" ("Y Scale.Name Label.Text")) -> ()  [unwired: 2 in, 2 out]
        }
        frame #1 {
          w345 = u32 3 ("Legend:Number of Rows")
          n146 = property on="Level Lower Limit, dB" class="DigNum (strict)"() -> ("Value"=w334:dbl)  [unwired: 2 in, 2 out]
          n147 = property on="Freq Lower Limit, Hz" class="DigNum (strict)"() -> ("Value"=w338:dbl)  [unwired: 2 in, 2 out]
          n148 = property on="Freq Upper Limit, Hz" class="DigNum (strict)"() -> ("Value"=w337:dbl)  [unwired: 2 in, 2 out]
          n149 = Multiply(x=i8 22, y=w345) -> (x*y=w346:u32)
          n150 = Subtract(x=w340, y=w346) -> (x-y=w347:u32)
          n151 = property on="Current Spectrum" class="WFGraph (strict)"("Legend Visible"=TRUE ("Legend:Visible"), "PlotVisCheckbox"=TRUE ("Legend:Plot Visibility Checkbox Visible"), "LegNumRows"=w345, "LegLeft"=w341, "LegTop"=w347, "XScale.ScaleFit"=u8 0 ("X Scale.Scale Fit"), "YScale.ScaleFit"=u8 0 ("X Scale.Scale Fit"), "XScale.Minimum"=w338, "XScale.Maximum"=w337, "YScale.Maximum"=0.0 ("Y Scale.Range:Maximum"), "YScale.Minimum"=w334) -> ()  [unwired: 2 in, 2 out]
        }
      }
      n152 = flat-sequence "Current Plot Init" {
        tunnel: [w383] -> w246
        tunnel: [w382] -> w243
        tunnel: w246 -> [w398]
        tunnel: w243 -> [w397]
        frame #0 {
          w382 = 76 ("Position:Top")
          n153 = property on="Current Button" class="Bool (strict)"() -> ("Width"=w396:u32, "Left"=w395:i32)  [unwired: 2 in, 2 out]
          n154 = property on="Pane" class="Pane"() -> ("Width"=w392:u32, "Height"=w385:u32)  [unwired: 2 in, 2 out]
          n155 = property on="Current Amplitude Range" class="DigNum (strict)"() -> ("Value"=w380:dbl)  [unwired: 2 in, 2 out]
          n156 = Subtract(x=w392, y=u32 120) -> (x-y=w390:u32)
          n157 = Subtract(x=w385, y=u32 130) -> (x-y=w389:u32)
          n158 = Compound Arithmetic op=ADD(w396, w395, 10 ("value")) -> (w383:u32)
          n159 = Subtract(x=w390, y=w383) -> (x-y=w384:u32)
          n160 = Subtract(x=w389, y=w382) -> (x-y=w387:u32)
          n161 = Negate(x=w380) -> (-x=w381:dbl)
          n162 = property on="Current" class="WFGraph (strict)"("Left"=w383, "Top"=w382, "Height"=w387, "Width"=w384, "Visible"=TRUE, "YScale.ScaleFit"=u8 0 ("Y Scale.Scale Fit"), "YScale.Maximum"=w380, "YScale.Minimum"=w381, "YScale.NameLbl.Text"="Current, A" ("Y Scale.Name Label.Text"), "XScale.NameLbl.Text"="Time, s" ("X Scale.Name Label.Text")) -> ()  [unwired: 2 in, 2 out]
        }
        frame #1 {
          w401 = u32 3 ("Legend:Number of Rows")
          n163 = Multiply(x=i8 22, y=w401) -> (x*y=w400:u32)
          n164 = Subtract(x=w397, y=w400) -> (x-y=w399:u32)
          n165 = property on="Current" class="WFGraph (strict)"("Legend Visible"=TRUE ("Legend:Visible"), "PlotVisCheckbox"=TRUE ("Legend:Plot Visibility Checkbox Visible"), "LegNumRows"=w401, "LegLeft"=w398, "LegTop"=w399) -> ()  [unwired: 2 in, 2 out]
        }
      }
      n166 = flat-sequence "Voltage Plot Init" {
        tunnel: [w411] -> w245
        tunnel: [w409] -> w244
        tunnel: w245 -> [w426]
        tunnel: w244 -> [w424]
        frame #0 {
          w409 = 76 ("Position:Top")
          n167 = property on="Current Button" class="Bool (strict)"() -> ("Width"=w423:u32, "Left"=w422:i32)  [unwired: 2 in, 2 out]
          n168 = property on="Pane" class="Pane"() -> ("Width"=w419:u32, "Height"=w412:u32)  [unwired: 2 in, 2 out]
          n169 = property on="Voltage Amplitude Range" class="DigNum (strict)"() -> ("Value"=w408:dbl)  [unwired: 2 in, 2 out]
          n170 = Subtract(x=w419, y=u32 120) -> (x-y=w417:u32)
          n171 = Subtract(x=w412, y=u32 130) -> (x-y=w416:u32)
          n172 = Compound Arithmetic op=ADD(w423, w422, 10 ("value")) -> (w411:u32)
          n173 = Subtract(x=w417, y=w411) -> (x-y=w410:u32)
          n174 = Subtract(x=w416, y=w409) -> (x-y=w414:u32)
          n175 = Negate(x=w408) -> (-x=w407:dbl)
          n176 = property on="Voltage" class="WFGraph (strict)"("Left"=w411, "Top"=w409, "Height"=w414, "Width"=w410, "Visible"=FALSE, "YScale.ScaleFit"=u8 0 ("Y Scale.Scale Fit"), "YScale.Maximum"=w408, "YScale.Minimum"=w407, "YScale.NameLbl.Text"="Voltage, V" ("Y Scale.Name Label.Text"), "XScale.NameLbl.Text"="Time, s" ("X Scale.Name Label.Text")) -> ()  [unwired: 2 in, 2 out]
        }
        frame #1 {
          w430 = u32 3 ("Legend:Number of Rows")
          n177 = Multiply(x=i8 22, y=w430) -> (x*y=w431:u32)
          n178 = Subtract(x=w424, y=w431) -> (x-y=w432:u32)
          n179 = property on="Voltage" class="WFGraph (strict)"("Legend Visible"=TRUE ("Legend:Visible"), "PlotVisCheckbox"=TRUE ("Legend:Plot Visibility Checkbox Visible"), "LegNumRows"=w430, "LegLeft"=w426, "LegTop"=w432, "LegDisable"=FALSE ("Legend:Disable")) -> ()  [unwired: 2 in, 2 out]
        }
      }
    }
  }
  n180 = property class="DAQmx System"() -> ("DevNames"=w14:tag[])  [unwired: 2 in, 2 out]
  n181 = while {
    stop <- FALSE stop-if-true
    n182 = event shown="[12] \"Continious Log\": Value Change" {
      selector: _ -> [_ _ _ _ _ _ _ _ _ _ _ _ _ _ _ _]
      dyn-events: _ -> [_ _ _ _ _ _ _ _ _ _ _ _ _ _ _ _]
      timeout: _ -> [_ _ _ _ _ _ _ _ _ _ _ _ _ _ _ _]
      event Timeout {
        n183 = event-data() -> ()  [unwired: 1 in, 3 out]
      }
      event "Freq Upper Limit, Hz": Value Change {
        n184 = event-data() -> ("NewVal"=w434:dbl)  [unwired: 1 in]
        n185 = flat-sequence {
          tunnel: w434 -> [w439]
          frame #0 {
            n186 = property on="Freq Lower Limit, Hz" class="DigNum (strict)"() -> ("Value"=w438:dbl)  [unwired: 2 in, 2 out]
            n187 = Add(x=w438, y=10.0) -> (x+y=w435:dbl)
            n188 = Less?(x=w439, y=w435) -> (x < y?=w436:bool)
            n189 = case shown="True" w436 {
              tunnel: w435 -> [_ w440]
              frame False {
              }
              frame True {
                n190 = property on="Freq Upper Limit, Hz" class="DigNum (strict)"("Value"=w440) -> ()  [unwired: 2 in, 2 out]
              }
            }
          }
          frame #1 {
            n191 = property on="Freq Upper Limit, Hz" class="DigNum (strict)"() -> ("Value"=w441:dbl)  [unwired: 2 in, 2 out]
            n192 = property on="Current Spectrum" class="WFGraph (strict)"("XScale.Maximum"=w441) -> ()  [unwired: 2 in, 2 out]
            n193 = property on="Voltage Spectrum" class="WFGraph (strict)"("XScale.Maximum"=w441) -> ()  [unwired: 2 in, 2 out]
            n194 = property on="Park Spectrum" class="WFGraph (strict)"("XScale.Maximum"=w441) -> ()  [unwired: 2 in, 2 out]
          }
        }
      }
      event "Voltage Amplitude Range": Value Change {
        n195 = event-data() -> ("NewVal"=w443:dbl)  [unwired: 1 in]
        n196 = Negate(x=w443) -> (-x=w442:dbl)
        n197 = property on="Voltage" class="WFGraph (strict)"("YScale.Maximum"=w443, "YScale.Minimum"=w442) -> ()  [unwired: 2 in, 2 out]
      }
      event "Current Amplitude Range": Value Change {
        n198 = event-data() -> ("NewVal"=w444:dbl)  [unwired: 1 in]
        n199 = Negate(x=w444) -> (-x=w445:dbl)
        n200 = property on="Current" class="WFGraph (strict)"("YScale.Maximum"=w444, "YScale.Minimum"=w445) -> ()  [unwired: 2 in, 2 out]
      }
      event "Voltage Spectrum Button": Value Change {
        n201 = event-data() -> ("NewVal"=w446:bool)  [unwired: 1 in]
        n202 = case shown="True" w446 {
          frame False {
            n203 = property on="Voltage Spectrum Button" class="Bool (strict)"("Value"=TRUE ("Voltage Button")) -> ()  [unwired: 2 in, 2 out]
          }
          frame True {
            n204 = property on="Voltage" class="WFGraph (strict)"("Visible"=FALSE) -> ()  [unwired: 2 in, 2 out]
            n205 = property on="Godograph Button" class="Bool (strict)"("Value"=FALSE ("Visible")) -> ()  [unwired: 2 in, 2 out]
            n206 = property on="Voltage Button" class="Bool (strict)"("Value"=FALSE ("Visible")) -> ()  [unwired: 2 in, 2 out]
            n207 = property on="Current" class="WFGraph (strict)"("Visible"=FALSE) -> ()  [unwired: 2 in, 2 out]
            n208 = property on="Current Spectrum Button" class="Bool (strict)"("Value"=FALSE ("Visible")) -> ()  [unwired: 2 in, 2 out]
            n209 = property on="Park Spectrum Button" class="Bool (strict)"("Value"=FALSE ("Visible")) -> ()  [unwired: 2 in, 2 out]
            n210 = property on="Current Button" class="Bool (strict)"("Value"=FALSE ("Visible")) -> ()  [unwired: 2 in, 2 out]
            n211 = property on="Freq Lower Limit, Hz" class="DigNum (strict)"("Visible"=TRUE) -> ()  [unwired: 2 in, 2 out]
            n212 = property on="Current Amplitude Range" class="DigNum (strict)"("Visible"=FALSE) -> ()  [unwired: 2 in, 2 out]
            n213 = property on="Godograph" class="XYGraph (strict)"("Visible"=FALSE) -> ()  [unwired: 2 in, 2 out]
            n214 = property on="Voltage Spectrum" class="WFGraph (strict)"("Visible"=TRUE) -> ()  [unwired: 2 in, 2 out]
            n215 = property on="Level Lower Limit, dB" class="DigNum (strict)"("Visible"=TRUE) -> ()  [unwired: 2 in, 2 out]
            n216 = property on="Voltage Amplitude Range" class="DigNum (strict)"("Visible"=FALSE) -> ()  [unwired: 2 in, 2 out]
            n217 = property on="Current Spectrum" class="WFGraph (strict)"("Visible"=FALSE) -> ()  [unwired: 2 in, 2 out]
            n218 = property on="Park Spectrum" class="WFGraph (strict)"("Visible"=FALSE) -> ()  [unwired: 2 in, 2 out]
            n219 = property on="Freq Upper Limit, Hz" class="DigNum (strict)"("Visible"=TRUE) -> ()  [unwired: 2 in, 2 out]
          }
        }
      }
      event "Freq Lower Limit, Hz": Value Change {
        n220 = event-data() -> ("NewVal"=w464:dbl)  [unwired: 1 in]
        n221 = flat-sequence {
          tunnel: w464 -> [w469]
          frame #0 {
            n222 = property on="Freq Upper Limit, Hz" class="DigNum (strict)"() -> ("Value"=w468:dbl)  [unwired: 2 in, 2 out]
            n223 = Subtract(x=w468, y=10.0) -> (x-y=w465:dbl)
            n224 = Greater?(x=w469, y=w465) -> (0:w466:bool)
            n225 = case shown="True" w466 {
              tunnel: w465 -> [_ w470]
              frame False {
              }
              frame True {
                n226 = property on="Freq Lower Limit, Hz" class="DigNum (strict)"("Value"=w470) -> ()  [unwired: 2 in, 2 out]
              }
            }
          }
          frame #1 {
            n227 = property on="Freq Lower Limit, Hz" class="DigNum (strict)"() -> ("Value"=w471:dbl)  [unwired: 2 in, 2 out]
            n228 = property on="Current Spectrum" class="WFGraph (strict)"("XScale.Minimum"=w471) -> ()  [unwired: 2 in, 2 out]
            n229 = property on="Voltage Spectrum" class="WFGraph (strict)"("XScale.Minimum"=w471) -> ()  [unwired: 2 in, 2 out]
            n230 = property on="Park Spectrum" class="WFGraph (strict)"("XScale.Minimum"=w471) -> ()  [unwired: 2 in, 2 out]
          }
        }
      }
      event "Level Lower Limit, dB": Value Change {
        n231 = event-data() -> ("NewVal"=w472:dbl)  [unwired: 1 in]
        n232 = flat-sequence {
          tunnel: w472 -> [w473]
          frame #0 {
            w474 = -10.0 ("y")
            n233 = Greater?(x=w473, y=w474) -> (0:w475:bool)
            n234 = Select(t=w474, s=w475, f=w473) -> (s? t:f=w476:dbl)
            n235 = property on="Level Lower Limit, dB" class="DigNum (strict)"("Value"=w476) -> ()  [unwired: 2 in, 2 out]
          }
          frame #1 {
            n236 = property on="Level Lower Limit, dB" class="DigNum (strict)"() -> ("Value"=w477:dbl)  [unwired: 2 in, 2 out]
            n237 = property on="Current Spectrum" class="WFGraph (strict)"("YScale.Minimum"=w477) -> ()  [unwired: 2 in, 2 out]
            n238 = property on="Voltage Spectrum" class="WFGraph (strict)"("YScale.Minimum"=w477) -> ()  [unwired: 2 in, 2 out]
            n239 = property on="Park Spectrum" class="WFGraph (strict)"("YScale.Minimum"=w477) -> ()  [unwired: 2 in, 2 out]
          }
        }
      }
      event "Current Spectrum Button": Value Change {
        n240 = event-data() -> ("NewVal"=w478:bool)  [unwired: 1 in]
        n241 = case shown="True" w478 {
          frame False {
            n242 = property on="Current Spectrum Button" class="Bool (strict)"("Value"=TRUE ("Voltage Button")) -> ()  [unwired: 2 in, 2 out]
          }
          frame True {
            n243 = property on="Voltage" class="WFGraph (strict)"("Visible"=FALSE) -> ()  [unwired: 2 in, 2 out]
            n244 = property on="Freq Upper Limit, Hz" class="DigNum (strict)"("Visible"=TRUE) -> ()  [unwired: 2 in, 2 out]
            n245 = property on="Current Button" class="Bool (strict)"("Value"=FALSE ("Visible")) -> ()  [unwired: 2 in, 2 out]
            n246 = property on="Current" class="WFGraph (strict)"("Visible"=FALSE) -> ()  [unwired: 2 in, 2 out]
            n247 = property on="Voltage Spectrum Button" class="Bool (strict)"("Value"=FALSE ("Visible")) -> ()  [unwired: 2 in, 2 out]
            n248 = property on="Voltage Button" class="Bool (strict)"("Value"=FALSE ("Visible")) -> ()  [unwired: 2 in, 2 out]
            n249 = property on="Godograph Button" class="Bool (strict)"("Value"=FALSE ("Visible")) -> ()  [unwired: 2 in, 2 out]
            n250 = property on="Park Spectrum Button" class="Bool (strict)"("Value"=FALSE ("Visible")) -> ()  [unwired: 2 in, 2 out]
            n251 = property on="Godograph" class="XYGraph (strict)"("Visible"=FALSE) -> ()  [unwired: 2 in, 2 out]
            n252 = property on="Current Amplitude Range" class="DigNum (strict)"("Visible"=FALSE) -> ()  [unwired: 2 in, 2 out]
            n253 = property on="Freq Lower Limit, Hz" class="DigNum (strict)"("Visible"=TRUE) -> ()  [unwired: 2 in, 2 out]
            n254 = property on="Voltage Spectrum" class="WFGraph (strict)"("Visible"=FALSE) -> ()  [unwired: 2 in, 2 out]
            n255 = property on="Voltage Amplitude Range" class="DigNum (strict)"("Visible"=FALSE) -> ()  [unwired: 2 in, 2 out]
            n256 = property on="Current Spectrum" class="WFGraph (strict)"("Visible"=TRUE) -> ()  [unwired: 2 in, 2 out]
            n257 = property on="Park Spectrum" class="WFGraph (strict)"("Visible"=FALSE) -> ()  [unwired: 2 in, 2 out]
            n258 = property on="Level Lower Limit, dB" class="DigNum (strict)"("Visible"=TRUE) -> ()  [unwired: 2 in, 2 out]
          }
        }
      }
      event "Godograph Button": Value Change {
        n259 = event-data() -> ("NewVal"=w496:bool)  [unwired: 1 in]
        n260 = case shown="True" w496 {
          frame False {
            n261 = property on="Godograph Button" class="Bool (strict)"("Value"=TRUE ("Voltage Button")) -> ()  [unwired: 2 in, 2 out]
          }
          frame True {
            n262 = property on="Voltage" class="WFGraph (strict)"("Visible"=FALSE) -> ()  [unwired: 2 in, 2 out]
            n263 = property on="Level Lower Limit, dB" class="DigNum (strict)"("Visible"=FALSE) -> ()  [unwired: 2 in, 2 out]
            n264 = property on="Current Button" class="Bool (strict)"("Value"=FALSE ("Visible")) -> ()  [unwired: 2 in, 2 out]
            n265 = property on="Current" class="WFGraph (strict)"("Visible"=FALSE) -> ()  [unwired: 2 in, 2 out]
            n266 = property on="Voltage Spectrum Button" class="Bool (strict)"("Value"=FALSE ("Visible")) -> ()  [unwired: 2 in, 2 out]
            n267 = property on="Freq Lower Limit, Hz" class="DigNum (strict)"("Visible"=FALSE) -> ()  [unwired: 2 in, 2 out]
            n268 = property on="Freq Upper Limit, Hz" class="DigNum (strict)"("Visible"=FALSE) -> ()  [unwired: 2 in, 2 out]
            n269 = property on="Current Spectrum Button" class="Bool (strict)"("Value"=FALSE ("Visible")) -> ()  [unwired: 2 in, 2 out]
            n270 = property on="Park Spectrum Button" class="Bool (strict)"("Value"=FALSE ("Visible")) -> ()  [unwired: 2 in, 2 out]
            n271 = property on="Godograph" class="XYGraph (strict)"("Visible"=TRUE) -> ()  [unwired: 2 in, 2 out]
            n272 = property on="Current Amplitude Range" class="DigNum (strict)"("Visible"=FALSE) -> ()  [unwired: 2 in, 2 out]
            n273 = property on="Voltage Spectrum" class="WFGraph (strict)"("Visible"=FALSE) -> ()  [unwired: 2 in, 2 out]
            n274 = property on="Voltage Amplitude Range" class="DigNum (strict)"("Visible"=FALSE) -> ()  [unwired: 2 in, 2 out]
            n275 = property on="Voltage Button" class="Bool (strict)"("Value"=FALSE ("Visible")) -> ()  [unwired: 2 in, 2 out]
            n276 = property on="Park Spectrum" class="WFGraph (strict)"("Visible"=FALSE) -> ()  [unwired: 2 in, 2 out]
            n277 = property on="Current Spectrum" class="WFGraph (strict)"("Visible"=FALSE) -> ()  [unwired: 2 in, 2 out]
          }
        }
      }
      event "Voltage Button": Value Change {
        n278 = event-data() -> ("NewVal"=w514:bool)  [unwired: 1 in]
        n279 = case shown="True" w514 {
          frame False {
            n280 = property on="Voltage Button" class="Bool (strict)"("Value"=TRUE ("Voltage Button")) -> ()  [unwired: 2 in, 2 out]
          }
          frame True {
            n281 = property on="Current" class="WFGraph (strict)"("Visible"=FALSE) -> ()  [unwired: 2 in, 2 out]
            n282 = property on="Godograph Button" class="Bool (strict)"("Value"=FALSE ("Visible")) -> ()  [unwired: 2 in, 2 out]
            n283 = property on="Voltage Spectrum Button" class="Bool (strict)"("Value"=FALSE ("Visible")) -> ()  [unwired: 2 in, 2 out]
            n284 = property on="Voltage" class="WFGraph (strict)"("Visible"=TRUE) -> ()  [unwired: 2 in, 2 out]
            n285 = property on="Freq Lower Limit, Hz" class="DigNum (strict)"("Visible"=FALSE) -> ()  [unwired: 2 in, 2 out]
            n286 = property on="Freq Upper Limit, Hz" class="DigNum (strict)"("Visible"=FALSE) -> ()  [unwired: 2 in, 2 out]
            n287 = property on="Current Spectrum Button" class="Bool (strict)"("Value"=FALSE ("Visible")) -> ()  [unwired: 2 in, 2 out]
            n288 = property on="Current Button" class="Bool (strict)"("Value"=FALSE ("Visible")) -> ()  [unwired: 2 in, 2 out]
            n289 = property on="Park Spectrum Button" class="Bool (strict)"("Value"=FALSE ("Visible")) -> ()  [unwired: 2 in, 2 out]
            n290 = property on="Current Spectrum" class="WFGraph (strict)"("Visible"=FALSE) -> ()  [unwired: 2 in, 2 out]
            n291 = property on="Park Spectrum" class="WFGraph (strict)"("Visible"=FALSE) -> ()  [unwired: 2 in, 2 out]
            n292 = property on="Current Amplitude Range" class="DigNum (strict)"("Visible"=FALSE) -> ()  [unwired: 2 in, 2 out]
            n293 = property on="Godograph" class="XYGraph (strict)"("Visible"=FALSE) -> ()  [unwired: 2 in, 2 out]
            n294 = property on="Voltage Spectrum" class="WFGraph (strict)"("Visible"=FALSE) -> ()  [unwired: 2 in, 2 out]
            n295 = property on="Voltage Amplitude Range" class="DigNum (strict)"("Visible"=TRUE) -> ()  [unwired: 2 in, 2 out]
            n296 = property on="Level Lower Limit, dB" class="DigNum (strict)"("Visible"=FALSE) -> ()  [unwired: 2 in, 2 out]
          }
        }
      }
      event "Current Button": Value Change {
        n297 = event-data() -> ("NewVal"=w532:bool)  [unwired: 1 in]
        n298 = case shown="True" w532 {
          frame False {
            n299 = property on="Current Button" class="Bool (strict)"("Value"=TRUE ("Visible")) -> ()  [unwired: 2 in, 2 out]
          }
          frame True {
            n300 = property on="Voltage" class="WFGraph (strict)"("Visible"=FALSE) -> ()  [unwired: 2 in, 2 out]
            n301 = property on="Godograph Button" class="Bool (strict)"("Value"=FALSE ("Visible")) -> ()  [unwired: 2 in, 2 out]
            n302 = property on="Voltage Spectrum Button" class="Bool (strict)"("Value"=FALSE ("Visible")) -> ()  [unwired: 2 in, 2 out]
            n303 = property on="Current" class="WFGraph (strict)"("Visible"=TRUE) -> ()  [unwired: 2 in, 2 out]
            n304 = property on="Voltage Button" class="Bool (strict)"("Value"=FALSE ("Visible")) -> ()  [unwired: 2 in, 2 out]
            n305 = property on="Level Lower Limit, dB" class="DigNum (strict)"("Visible"=FALSE) -> ()  [unwired: 2 in, 2 out]
            n306 = property on="Park Spectrum" class="WFGraph (strict)"("Visible"=FALSE) -> ()  [unwired: 2 in, 2 out]
            n307 = property on="Freq Upper Limit, Hz" class="DigNum (strict)"("Visible"=FALSE) -> ()  [unwired: 2 in, 2 out]
            n308 = property on="Current Spectrum Button" class="Bool (strict)"("Value"=FALSE ("Visible")) -> ()  [unwired: 2 in, 2 out]
            n309 = property on="Park Spectrum Button" class="Bool (strict)"("Value"=FALSE ("Visible")) -> ()  [unwired: 2 in, 2 out]
            n310 = property on="Voltage Spectrum" class="WFGraph (strict)"("Visible"=FALSE) -> ()  [unwired: 2 in, 2 out]
            n311 = property on="Current Amplitude Range" class="DigNum (strict)"("Visible"=TRUE) -> ()  [unwired: 2 in, 2 out]
            n312 = property on="Freq Lower Limit, Hz" class="DigNum (strict)"("Visible"=FALSE) -> ()  [unwired: 2 in, 2 out]
            n313 = property on="Voltage Amplitude Range" class="DigNum (strict)"("Visible"=FALSE) -> ()  [unwired: 2 in, 2 out]
            n314 = property on="Godograph" class="XYGraph (strict)"("Visible"=FALSE) -> ()  [unwired: 2 in, 2 out]
            n315 = property on="Current Spectrum" class="WFGraph (strict)"("Visible"=FALSE) -> ()  [unwired: 2 in, 2 out]
          }
        }
      }
      event "Park Spectrum Button": Value Change {
        n316 = event-data() -> ("NewVal"=w550:bool)  [unwired: 1 in]
        n317 = case shown="True" w550 {
          frame False {
            n318 = property on="Park Spectrum Button" class="Bool (strict)"("Value"=TRUE ("Visible")) -> ()  [unwired: 2 in, 2 out]
          }
          frame True {
            n319 = property on="Voltage" class="WFGraph (strict)"("Visible"=FALSE) -> ()  [unwired: 2 in, 2 out]
            n320 = property on="Level Lower Limit, dB" class="DigNum (strict)"("Visible"=TRUE) -> ()  [unwired: 2 in, 2 out]
            n321 = property on="Current Button" class="Bool (strict)"("Value"=FALSE ("Visible")) -> ()  [unwired: 2 in, 2 out]
            n322 = property on="Current" class="WFGraph (strict)"("Visible"=FALSE) -> ()  [unwired: 2 in, 2 out]
            n323 = property on="Voltage Button" class="Bool (strict)"("Value"=FALSE ("Visible")) -> ()  [unwired: 2 in, 2 out]
            n324 = property on="Voltage Spectrum Button" class="Bool (strict)"("Value"=FALSE ("Visible")) -> ()  [unwired: 2 in, 2 out]
            n325 = property on="Freq Lower Limit, Hz" class="DigNum (strict)"("Visible"=TRUE) -> ()  [unwired: 2 in, 2 out]
            n326 = property on="Freq Upper Limit, Hz" class="DigNum (strict)"("Visible"=TRUE) -> ()  [unwired: 2 in, 2 out]
            n327 = property on="Current Spectrum Button" class="Bool (strict)"("Value"=FALSE ("Visible")) -> ()  [unwired: 2 in, 2 out]
            n328 = property on="Current Spectrum" class="WFGraph (strict)"("Visible"=FALSE) -> ()  [unwired: 2 in, 2 out]
            n329 = property on="Current Amplitude Range" class="DigNum (strict)"("Visible"=FALSE) -> ()  [unwired: 2 in, 2 out]
            n330 = property on="Godograph Button" class="Bool (strict)"("Value"=FALSE ("Voltage Button")) -> ()  [unwired: 2 in, 2 out]
            n331 = property on="Voltage Amplitude Range" class="DigNum (strict)"("Visible"=FALSE) -> ()  [unwired: 2 in, 2 out]
            n332 = property on="Godograph" class="XYGraph (strict)"("Visible"=FALSE) -> ()  [unwired: 2 in, 2 out]
            n333 = property on="Park Spectrum" class="WFGraph (strict)"("Visible"=TRUE) -> ()  [unwired: 2 in, 2 out]
            n334 = property on="Voltage Spectrum" class="WFGraph (strict)"("Visible"=FALSE) -> ()  [unwired: 2 in, 2 out]
          }
        }
      }
      event "Continious Log": Value Change {
        n335 = event-data() -> ()  [unwired: 1 in, 1 out]
        n336 = property on="Continious Log Flag" class="Bool (strict)"() -> ("Value"=w568:bool)  [unwired: 2 in, 2 out]
        n337 = case shown="False" w568 {
          frame False {
            n338 = property on="Continious Log Flag" class="Bool (strict)"("Value"=TRUE ("Continious Log Flag")) -> ()  [unwired: 2 in, 2 out]
            n339 = property on="Start Log" class="Bool (strict)"("DisabledEnum"=T5."Disabled and Grayed Out" ("Disabled")) -> ()  [unwired: 2 in, 2 out]
            n340 = property on="Continious Log" class="Bool (strict)"("BoolText.Text"="Stop\nContinuous\nLog" ("Boolean Text.Text"), "Value"=FALSE ("Continious Log Flag")) -> ()  [unwired: 2 in, 2 out]
            n341 = property on="Counter" class="DigNum (strict)"("Visible"=TRUE, "Value"=0.0 ("Counter")) -> ()  [unwired: 2 in, 2 out]
          }
          frame True {
            n342 = property on="Continious Log Flag" class="Bool (strict)"("Value"=FALSE ("Continious Log Flag")) -> ()  [unwired: 2 in, 2 out]
            n343 = property on="Start Log" class="Bool (strict)"("DisabledEnum"=T5."Enabled" ("Disabled")) -> ()  [unwired: 2 in, 2 out]
            n344 = property on="Counter" class="DigNum (strict)"("Visible"=FALSE) -> ()  [unwired: 2 in, 2 out]
            n345 = property on="Continious Log" class="Bool (strict)"("BoolText.Text"="Start\nContinuous\nLog" ("Boolean Text.Text"), "Value"=FALSE ("Continious Log Flag")) -> ()  [unwired: 2 in, 2 out]
          }
        }
      }
      event Pane Size {
        n346 = event-data() -> ()  [unwired: 1 in, 1 out]
        n347 = property on="Pane" class="Pane"() -> ("Width"=w581:u32, "Height"=w580:u32)  [unwired: 2 in, 2 out]
        n348 = stacked-sequence {
          tunnel: w581 -> [w583 w593 w604 w615 w626 w641 w661]
          tunnel: w580 -> [w592 w594 w605 w616 w627 w642 w662]
          frame #0 {
            n349 = property on="Current Button" class="Bool (strict)"() -> ("Width"=w589:u32, "Left"=w588:i32)  [unwired: 2 in, 2 out]
            n350 = Subtract(x=w583, y=u32 120) -> (x-y=w585:u32)
            n351 = Compound Arithmetic op=ADD(w589, w588, 10 ("value")) -> (w584:u32)
            n352 = Subtract(x=w585, y=w584) -> (x-y=w582:u32)
            n353 = Subtract(x=w592, y=u32 206) -> (x-y=w590:u32)
            n354 = property on="Voltage" class="WFGraph (strict)"("Height"=w590, "Width"=w582) -> ()  [unwired: 2 in, 2 out]
          }
          frame #1 {
            n355 = property on="Current Button" class="Bool (strict)"() -> ("Width"=w601:u32, "Left"=w600:i32)  [unwired: 2 in, 2 out]
            n356 = Subtract(x=w593, y=u32 120) -> (x-y=w597:u32)
            n357 = Compound Arithmetic op=ADD(w601, w600, 10 ("value")) -> (w596:u32)
            n358 = Subtract(x=w597, y=w596) -> (x-y=w595:u32)
            n359 = Subtract(x=w594, y=u32 206) -> (x-y=w602:u32)
            n360 = property on="Current" class="WFGraph (strict)"("Height"=w602, "Width"=w595) -> ()  [unwired: 2 in, 2 out]
          }
          frame #2 {
            n361 = property on="Current Button" class="Bool (strict)"() -> ("Width"=w612:u32, "Left"=w611:i32)  [unwired: 2 in, 2 out]
            n362 = Subtract(x=w604, y=u32 120) -> (x-y=w608:u32)
            n363 = Compound Arithmetic op=ADD(w612, w611, 10 ("value")) -> (w607:u32)
            n364 = Subtract(x=w608, y=w607) -> (x-y=w606:u32)
            n365 = Subtract(x=w605, y=u32 206) -> (x-y=w613:u32)
            n366 = property on="Current Spectrum" class="WFGraph (strict)"("Height"=w613, "Width"=w606) -> ()  [unwired: 2 in, 2 out]
          }
          frame #3 {
            n367 = property on="Current Button" class="Bool (strict)"() -> ("Width"=w623:u32, "Left"=w622:i32)  [unwired: 2 in, 2 out]
            n368 = Subtract(x=w615, y=u32 120) -> (x-y=w619:u32)
            n369 = Compound Arithmetic op=ADD(w623, w622, 10 ("value")) -> (w618:u32)
            n370 = Subtract(x=w619, y=w618) -> (x-y=w617:u32)
            n371 = Subtract(x=w616, y=u32 206) -> (x-y=w624:u32)
            n372 = property on="Voltage Spectrum" class="WFGraph (strict)"("Height"=w624, "Width"=w617) -> ()  [unwired: 2 in, 2 out]
          }
          frame #4 {
            n373 = property on="Current Button" class="Bool (strict)"() -> ("Width"=w634:u32, "Left"=w633:i32)  [unwired: 2 in, 2 out]
            n374 = Subtract(x=w626, y=u32 120) -> (x-y=w630:u32)
            n375 = Compound Arithmetic op=ADD(w634, w633, 10 ("value")) -> (w629:u32)
            n376 = Subtract(x=w630, y=w629) -> (x-y=w628:u32)
            n377 = Subtract(x=w627, y=u32 186) -> (x-y=w635:u32)
            n378 = property on="Park Spectrum" class="WFGraph (strict)"("Height"=w635, "Width"=w628) -> ()  [unwired: 2 in, 2 out]
          }
          frame #5 {
            n379 = property on="Current Button" class="Bool (strict)"() -> ("Width"=w649:u32, "Left"=w648:i32)  [unwired: 2 in, 2 out]
            n380 = Subtract(x=w641, y=u32 120) -> (x-y=w647:u32)
            n381 = Compound Arithmetic op=ADD(w649, w648, 10 ("value")) -> (w646:u32)
            n382 = Subtract(x=w647, y=w646) -> (x-y=w638:u32)
            n383 = Subtract(x=w642, y=u32 186) -> (x-y=w639:u32)
            n384 = Less?(x=w639, y=w638) -> (x < y?=w640:bool)
            n385 = Select(t=w639, s=w640, f=w638) -> (s? t:f=w637:u32)
            n386 = property on="Godograph" class="XYGraph (strict)"("Height"=w637, "Width"=w637) -> ()  [unwired: 2 in, 2 out]
          }
          frame #6 {
            n387 = Divide(x=w661, y=u32 2) -> (x/y=w664:dbl)
            n388 = property on="Experiment Name" class="Str"() -> ("Width"=w653:u32)  [unwired: 2 in, 2 out]
            n389 = property on="Start Log" class="Bool (strict)"() -> ("Height"=w670:u32, "Width"=w651:u32)  [unwired: 2 in, 2 out]
            n390 = Add(x=w670, y=u32 10) -> (x+y=w668:u32)
            n391 = Compound Arithmetic op=ADD(w651, w653, u32 10 ("value")) -> (w650:u32)
            n392 = Subtract(x=w662, y=w668) -> (x-y=w667:u32)
            n393 = Divide(x=w650, y=u32 2) -> (x/y=w663:dbl)
            n394 = Subtract(x=w664, y=w663) -> (x-y=w655:dbl)
            n395 = property on="Start Log" class="Bool (strict)"("Left"=w655, "Top"=w667) -> ("Top"=w660:i32, "Width"=w657:u32)  [unwired: 2 in, 2 out]
            n396 = Add(x=w660, y=5) -> (x+y=w658:i32)
            n397 = Compound Arithmetic op=ADD(w657, u32 10 ("value"), w655) -> (w654:dbl)
            n398 = property on="Experiment Name" class="Str"("Left"=w654, "Top"=w658) -> ()  [unwired: 2 in, 2 out]
          }
        }
      }
      event "Experiment Name": Value Change {
        n399 = event-data() -> ("NewVal"=w677:string)  [unwired: 1 in]
        n400 = Build Array (concatenate)(string[] ["\\", "/", ":", "*", "?", "\"", "<", ">", "|"], "\r", "\n") -> (w673:string[])
        n401 = for {
          tunnel: w673 -> [w681] mode=indexing
          shift-right: [w682] -> w675
          shift-left: w677 -> [w683]
          n402 = Search and Replace String(replace all?=TRUE ("replace all? (F)"), input string=w683, search string=w681) -> (result string=w682:string)  [unwired: 5 in, 3 out]
        }
        n403 = call <vilib>:"Trim Whitespace.vi"("string"=w675) -> ("trimmed string"=w676:string)  [unwired: 1 in]
        n404 = String Length(string=w676) -> (length=w679:i32)
        n405 = Equal To 0?(x=w679) -> (x = 0?=w678:bool)
        n406 = case shown="False" w678 {
          tunnel: w675 -> [w684 _]
          frame False {
            n407 = property on="Experiment Name" class="Str"("Value"=w684) -> ()  [unwired: 2 in, 2 out]
          }
          frame True {
            n408 = property on="Experiment Name" class="Str"("Value"="Unnamed" ("Experiment Name")) -> ()  [unwired: 2 in, 2 out]
          }
        }
      }
      event "Start Log": Value Change {
        n409 = event-data() -> ("NewVal"=w686:bool)  [unwired: 1 in]
        n410 = case shown="True" w686 {
          frame False {
            n411 = property on="Start Log" class="Bool (strict)"("Value"=TRUE ("Start Log")) -> ()  [unwired: 2 in, 2 out]
          }
          frame True {
            n412 = property on="Log flag" class="Bool (strict)"() -> ("Value"=w688:bool)  [unwired: 2 in, 2 out]
            n413 = case shown="False" w688 {
              frame False {
                n414 = property on="Log flag" class="Bool (strict)"("Value"=TRUE ("Log flag")) -> ()  [unwired: 2 in, 2 out]
              }
              frame True {
              }
            }
          }
        }
      }
    }
  }
  n415 = while {
    stop <- FALSE stop-if-true
    n416 = property on="Continious Log Flag" class="Bool (strict)"() -> ("Value"=w690:bool)  [unwired: 2 in, 2 out]
    n417 = case shown="True" w690 {
      frame False {
      }
      frame True {
        n418 = property on="Log flag" class="Bool (strict)"() -> ("Value"=w692:bool)  [unwired: 2 in, 2 out]
        n419 = case shown="False" w692 {
          frame False {
            n420 = flat-sequence {
              frame #0 {
                n421 = Wait (ms)(milliseconds to wait=u32 1000) -> ()  [unwired: 1 out]
              }
              frame #1 {
                n422 = property on="Log flag" class="Bool (strict)"("Value"=TRUE ("Log flag")) -> ()  [unwired: 2 in, 2 out]
              }
            }
          }
          frame True {
          }
        }
      }
    }
  }
  n423 = for {
    tunnel: w14 -> [w696] mode=indexing
    tunnel: [w695] -> w12 mode=indexing
    n424 = xnode "Match Regular Expression"("input string"=w696, "regular expression"="^Dev\\d$") -> ("whole match"=w695:string)  [unwired: 4 in, 4 out]
  }
  n425 = Array Size(array=w12) -> (size(s)=w13:i32)
  n426 = case shown="1.." w13 {
    tunnel: w12 -> [_ w815]
    tunnel: [_ w814] -> w2
    frame 0, Default {
      n427 = One Button Dialog(message="There is no DAQmx device") -> (true=w812:bool)  [unwired: 1 in]
      n428 = Stop(stop? (T)=w812) -> ()
    }
    frame 1.. {
      n429 = Index Array(array=w815) -> (element=w814:string)  [unwired: 1 in]
    }
  }
  n430 = Concatenate Strings(w2, "/ai3" ("string")) -> (w8:string)
  n431 = Concatenate Strings(w2, "/ai11" ("string")) -> (w7:string)
  n432 = Concatenate Strings(w2, "/ai12" ("string")) -> (w6:string)
  n433 = Build Array(w8, w7, w6) -> (w5:string[])
  n434 = call <vilib>:"DAQmx Flatten Channel String.vi"("names in"=w5) -> ("names out"=w4:string)  [unwired: 13 in, 1 out]
  n435 = Concatenate Strings(w2, "/ai0:2" ("string")) -> (w1:string)
  n436 = call-poly <vilib>:"DAQmx Create Virtual Channel.vi"("input terminal configuration"=w30, "physical channels"=w4, "name to assign"="Current") -> ("task out"=w29:refnum<k21>)  [unwired: 11 in, 1 out]
  n437 = call-poly <vilib>:"DAQmx Create Virtual Channel.vi"("task in"=w29, "input terminal configuration"=w31, "physical channels"=w1, "name to assign"="Voltage") -> ("task out"=w28:refnum<k21>)  [unwired: 10 in, 1 out]
  n438 = call-poly <vilib>:"DAQmx Timing.vi"("task/channels in"=w28, "sample mode"=w27, "rate"=w16) -> ("task out"=w26:refnum<k21>)  [unwired: 11 in, 1 out]
  n439 = Obtain Queue(name (unnamed)="Instatnt View", element data type=waveform(dbl)[] []) -> (queue out=w20:refnum<queue>)  [unwired: 3 in, 2 out]
  n440 = Obtain Queue(name (unnamed)="Logger", element data type=waveform(dbl)[] []) -> (queue out=w15:refnum<queue>)  [unwired: 3 in, 2 out]
  n441 = Divide(x=w16, y=10.0) -> (x/y=w22:dbl)
  n442 = while {
    tunnel: w20 -> [w833]
    stop <- FALSE stop-if-true
    n443 = Dequeue Element(queue=w833) -> (queue out=w831:refnum<queue>, element=w832:waveform(dbl)[])  [unwired: 2 in, 2 out]
    n444 = while {
      tunnel: w831 -> [w854]
      shift-right: [w852] -> w836
      shift-left: w832 -> [w851]
      i -> [w847]
      stop <- w848 stop-if-true
      n445 = Dequeue Element(queue=w854) -> (element=w853:waveform(dbl)[])  [unwired: 2 in, 3 out]
      n446 = Add(x=w847, y=2) -> (x+y=w845:i32)
      n447 = for {
        tunnel: w853 -> [w856] mode=indexing
        tunnel: [w855] -> w852 mode=indexing
        tunnel: w851 -> [w857] mode=indexing
        n448 = call-poly <vilib>:"Append Waveforms.vi"("waveform B"=w856, "waveform A"=w857) -> ("waveform out"=w855:waveform(dbl))  [unwired: 8 in, 1 out]
      }
      n449 = Multiply(x=w845, y=0.1) -> (x*y=w844:dbl)
      n450 = Add(x=w844, y=0.05) -> (x+y=w842:dbl)
      n451 = Greater Or Equal?(x=w842, y="Plot length , sec") -> (x >= y?=w848:bool)
    }
    n452 = call "Divide signals.vi"("All data"=w836) -> ("Voltages"=w835:waveform(dbl)[], "Currents"=w834:waveform(dbl)[])
    "Voltage" <- w835
    "Current" <- w834
    n453 = call "Build Spectrums.vi"("Waveforms"=w835) -> ("Spectrums"=→"Voltage Spectrum":waveform(dbl)[])
    n454 = call "ABC2DQ.vi"("ABC"=w835, "Waveform Name"="Voltage") -> ("d"=w840:waveform(dbl), "q"=w839:waveform(dbl), "Park Vector ^2"=w823:waveform(dbl))
    n455 = call "ABC2DQ.vi"("ABC"=w834, "Waveform Name"="Current") -> ("d"=w827:waveform(dbl), "q"=w826:waveform(dbl), "Park Vector ^2"=w822:waveform(dbl))
    n456 = call "Build Spectrums.vi"("Waveforms"=w834) -> ("Spectrums"=→"Current Spectrum":waveform(dbl)[])
    n457 = Unbundle By Name(w840) -> ("Y"=w838:dbl[])
    n458 = Unbundle By Name(w839) -> ("Y"=w837:dbl[])
    n459 = Unbundle By Name(w827) -> ("Y"=w828:dbl[])
    n460 = Unbundle By Name(w826) -> ("Y"=w829:dbl[])
    n461 = Build Array(w823, w822) -> (w819:waveform(dbl)[])
    n462 = Bundle("Y"=w838, "Y"=w837) -> (w830:cluster{"Y":dbl[], "Y":dbl[]})  [unwired: 1 in]
    n463 = Bundle("Y"=w828, "Y"=w829) -> (w825:cluster{"Y":dbl[], "Y":dbl[]})  [unwired: 1 in]
    n464 = call "Build Spectrums.vi"("Waveforms"=w819) -> ("Spectrums"=→"Park Spectrum":waveform(dbl)[])
    n465 = Build Array(w830, w825) -> (→"Godograph":cluster{"Y":dbl[], "Y":dbl[]}[])
  }
  n466 = while {
    tunnel: w26 -> [w873]
    tunnel: w22 -> [w871]
    tunnel: w20 -> [w870]
    tunnel: w15 -> [w859]
    stop <- FALSE stop-if-true
    n467 = call-poly <vilib>:"DAQmx Read.vi"("task/channels in"=w873, "number of samples per channel"=w871) -> ("data"=w869:waveform(dbl)[])  [unwired: 11 in, 2 out]
    n468 = call "Divide signals.vi"("All data"=w869) -> ("Voltages"=w867:waveform(dbl)[], "Currents"=w863:waveform(dbl)[])
    n469 = Subtract(x=w863, y=2.5 ("rate")) -> (x-y=w864:waveform(dbl)[])
    n470 = Multiply(x=w867, y=145.8 ("rate")) -> (x*y=w861:waveform(dbl)[])
    n471 = Multiply(x=w864, y=38.462 ("rate")) -> (x*y=w862:waveform(dbl)[])
    n472 = Insert Into Array(array=w862, new element=w861) -> (w858:waveform(dbl)[])  [unwired: 1 in]
    n473 = property on="Log flag" class="Bool (strict)"() -> ("Value"=w860:bool)  [unwired: 2 in, 2 out]
    n474 = Enqueue Element(queue=w870, element=w858) -> ()  [unwired: 2 in, 3 out]
    n475 = case shown="True" w860 {
      tunnel: w859 -> [_ w875]
      tunnel: w858 -> [_ w874]
      frame False {
      }
      frame True {
        n476 = Enqueue Element(queue=w875, element=w874) -> ()  [unwired: 2 in, 3 out]
      }
    }
  }
  n477 = while {
    tunnel: w15 -> [w885]
    stop <- FALSE stop-if-true
    n478 = Dequeue Element(queue=w885) -> (queue out=w884:refnum<queue>, element=w883:waveform(dbl)[])  [unwired: 2 in, 2 out]
    n479 = flat-sequence {
      tunnel: w883 -> [w929]
      tunnel: w884 -> [w930]
      tunnel: [w930] -> w882
      tunnel: [w929] -> w881
      tunnel: [w926] -> w880
      tunnel: [w939] -> w879
      tunnel: [w938] -> w911
      tunnel: [w937] -> w888
      tunnel: w882 -> [w936]
      tunnel: w881 -> [w935]
      frame #0 {
        n480 = property on="Experiment Name" class="Str"() -> ("Value"=w922:string)  [unwired: 2 in, 2 out]
        n481 = call <vilib>:"Application Directory.vi"() -> ("Application Directory"=w925:path)
        n482 = Build Path(base path=w925, name or relative path=path "Logs") -> (appended path=w923:path)
        n483 = Build Path(base path=w923, name or relative path=w922) -> (appended path=w916:path)
        n484 = call <vilib>:"Check if File or Folder Exists.vi"("path"=w916) -> ("file or folder exists?"=w917:bool)  [unwired: 8 in, 2 out]
        n485 = case shown="True" w917 {
          tunnel: w916 -> [w932 w933]
          tunnel: [w931 w933] -> w915
          frame False {
            n486 = Create Folder(path (use dialog)=w932) -> (created path=w931:path)  [unwired: 2 in, 2 out]
          }
          frame True {
          }
        }
        n487 = Get Date/Time In Seconds() -> (seconds since 1Jan1904=w921:timestamp)
        n488 = Format Date/Time String(time format string (%c)="%Y.%m.%d_%H-%M-%S.tdms", seconds (now)=w921) -> (date/time string=w919:string)  [unwired: 1 in]
        n489 = Build Path(base path=w915, name or relative path=w919) -> (appended path=w918:path)
        n490 = TDMS Open(5:FALSE ("create index file? (T)"), 10:T6."create or replace" ("operation (0:open)"), 11:w918) -> (3:w926:refnum<k34>)  [unwired: 4 in, 1 out]
      }
      frame #1 {
        n491 = while {
          shift-right: [w954] -> w938
          shift-left: w935 -> [w953]
          tunnel: [FALSE] -> w934
          tunnel: [w943] -> w939
          tunnel: [FALSE] -> w937
          tunnel: w936 -> [w940]
          i -> [w950]
          stop <- w951 stop-if-true
          n492 = Dequeue Element(queue=w940) -> (queue out=w943:refnum<queue>, element=w955:waveform(dbl)[])  [unwired: 2 in, 2 out]
          n493 = Add(x=w950, y=2) -> (x+y=w948:i32)
          n494 = for {
            tunnel: w955 -> [w957] mode=indexing
            tunnel: [w956] -> w954 mode=indexing
            tunnel: w953 -> [w958] mode=indexing
            n495 = call-poly <vilib>:"Append Waveforms.vi"("waveform B"=w957, "waveform A"=w958) -> ("waveform out"=w956:waveform(dbl))  [unwired: 8 in, 1 out]
          }
          n496 = Multiply(x=w948, y=0.1) -> (x*y=w947:dbl)
          n497 = Add(x=w947, y=0.05) -> (x+y=w945:dbl)
          n498 = Greater Or Equal?(x=w945, y="Log length, sec") -> (x >= y?=w951:bool)
        }
        n499 = property on="Log flag" class="Bool (strict)"("Value"=w934) -> ()  [unwired: 2 in, 2 out]
      }
    }
    n500 = property on="Start Log" class="Bool (strict)"("Value"=w888) -> ()  [unwired: 2 in, 2 out]
    n501 = call "Divide signals.vi"("All data"=w911) -> ("Voltages"=w906:waveform(dbl)[], "Currents"=w905:waveform(dbl)[])
    n502 = Dequeue Element(queue=w879, timeout in ms (-1)=1000) -> ()  [unwired: 1 in, 4 out]
    n503 = call "Build Spectrums.vi"("Waveforms"=w906) -> ("Spectrums"=w893:waveform(dbl)[])
    n504 = call "Build Spectrums.vi"("Waveforms"=w905) -> ("Spectrums"=w892:waveform(dbl)[])
    n505 = call "ABC2DQ.vi"("ABC"=w906, "Waveform Name"="Voltage") -> ("d"=w910:waveform(dbl), "q"=w909:waveform(dbl), "Park Vector ^2"=w904:waveform(dbl))
    n506 = call "ABC2DQ.vi"("ABC"=w905, "Waveform Name"="Current") -> ("d"=w908:waveform(dbl), "q"=w907:waveform(dbl), "Park Vector ^2"=w901:waveform(dbl))
    n507 = Insert Into Array "Time-Domain"(array=w906, new element #1=w910, new element #2=w909, new element #3=w905, new element #4=w908, new element #5=w907) -> (w898:waveform(dbl)[])  [unwired: 1 in]
    n508 = Build Array(w904) -> (w903:waveform(dbl)[])
    n509 = Build Array(w901) -> (w902:waveform(dbl)[])
    n510 = call "Build Spectrums.vi"("Waveforms"=w903) -> ("Spectrums"=w891:waveform(dbl)[])
    n511 = call "Build Spectrums.vi"("Waveforms"=w902) -> ("Spectrums"=w890:waveform(dbl)[])
    n512 = TDMS Write(0:w880, 5:"Time-Domain" ("group name in (Untitled)"), 7:string[] ["Ua", "Ub", "Uc", "Ud", "Uq", "Ia", "Ib", "Ic", "Id", "Iq"] ("channel name(s) in (Untitled)"), 9:w898) -> (4:w897:refnum<k34>)  [unwired: 2 in, 3 out]
    n513 = Insert Into Array "Frequency-Domain"(array=w893, new element #1=w892, new element #2=w891, new element #3=w890) -> (w889:waveform(dbl)[])  [unwired: 1 in]
    n514 = TDMS Write(0:w897, 5:"Frequency-Domain" ("group name in (Untitled)"), 7:string[] ["Ua", "Ub", "Uc", "Ia", "Ib", "Ic", "U_Park", "I_Park"] ("channel name(s) in (Untitled)"), 9:w889) -> (4:w894:refnum<k34>)  [unwired: 2 in, 3 out]
    n515 = property on="Continious Log Flag" class="Bool (strict)"() -> ("Value"=w876:bool)  [unwired: 2 in, 2 out]
    n516 = TDMS Close(11:w894) -> (3:w877:path)  [unwired: 1 in, 1 out]
    n517 = case shown="True" w876 {
      tunnel: w877 -> [_ _]
      frame False {
      }
      frame True {
        n518 = property on="Counter" class="DigNum (strict)"() -> ("Value"=w914:dbl)  [unwired: 2 in, 2 out]
        n519 = Increment(x=w914) -> (x+1=w913:dbl)
        n520 = property on="Counter" class="DigNum (strict)"("Value"=w913) -> ()  [unwired: 2 in, 2 out]
      }
    }
  }
